vi "app - Kim Thing -- torque.vi"() -> ()   [LabVIEW 2012]
uses:
  <vilib>/event_ctls.llb/eventvkey.ctl
  cursor winow.ctl
  polynomial - bilinear.ctl
  torque transformation selector.ctl
  countdown control.ctl
  cursor window action.ctl
  hash action control.ctl
  container action.ctl
  array -- fit control .ctl
  cursor action.ctl
  fit function selector control.ctl
  file -- read-write control.ctl
  torque -- filename action.ctl
  torque -- hash key.ctl
panel:
  in  "torque transformations":T1
  out "offset (deg)":dbl
  out "sin2theta fit":dbl[](array[numeric])
  out "Plot: slope vs angle":cluster{dbl[], dbl[]}[](graph)
  in  "main folder":path=path "C:/Users/224586/Downloads/arkady/Torque-Jun2013"
  in  "Tab : other":enum32{"indicators", "other", "slope fit"}(tab)
  out "Torque (a.u)":dbl
  out "field (T)":dbl
  in  "angle":u16(ring) items=["-54", "-36", "-9", "27", "36", "45", "54"]
  in  "temperature":u16(ring) items=["2K", "15K", "30K", "38K", "42K", "45K", "52K", "60K", "75K", "90K", "100K", "120K", "150K", "180K", "240K"]
  out "time (sec)":dbl=513.2382892057026
  in  "open (o)":bool
  in  "plot (p)":bool
  out "temperature (K)":dbl=369.642
  out "angle (deg)":dbl
  in  "rotation set":u16(ring) items=["rotationset1", "rotationset2", "rotationset3", "rotationset4", "rotationset5", "rotationset6"]
  in  "filename":u16(ring) items=["5_60K_-54.dat", "5_60K_-36.dat", "5_60K_-9.dat", "5_60K_27.dat", "5_60K_36.dat", "5_60K_45.dat", "5_60K_54.dat"]
  out "read OK":bool=TRUE
  out "Char":i16=46
  out "VKey":T2
  in  "Tab: timer":enum32{"timer ON", "timer OFF"}(tab)=enum."timer OFF"
  in  "timer  \"update\"":dbl(slide) min=-553366660.0 max=2129711151.0 step=0.010000000000000002 scale=0.0..100.0 scale format="%#3_3f"
  out "folder --OK":bool=TRUE
  in  "temperatures":dbl[](array[numeric])
  in  "plot type":T3(ring)=enum."plot vs Temperature"
  out "current angle  index":dbl=1431.5698546544484
  out "current time index":dbl=1431.5698546544484
  in  "angles (deg)":dbl[](array[numeric])
  in  "slopes":dbl[](array[numeric])
  out "slope fit parameters":dbl[](array[numeric])
  out "field offset":dbl=1431.5698546544484
  out "torque offset":dbl=1431.5698546544484
  out "right bound index":dbl=1431.5698546544484
  out "left bound index":dbl=1431.5698546544484
  in  "Tab : all":enum32{"everything", "everything else"}(tab)
  out "Plot: torque/field -- all":cluster{dbl[], dbl[]}[](graph)
  out "Plot: temp vs time":cluster{dbl[], dbl[]}[](graph)
  out "Plot: torque --one angle":cluster{dbl[], dbl[]}[](graph)
  out "Plot: field vs time":cluster{dbl[], dbl[]}[](graph)
  out "Plot: torque -- all angles":cluster{dbl[], dbl[]}[](graph)
  in  "file path":path=path "C:/Data/GloveBox/Pu-delta-temperature_experiment/4_Sweep_370K_114.59min/9w/monitor/381_mo.dat"
  in  "cursor bracket: torque -- all angles":T4={"left"=364.687, "right "=367.23699999999997, "center"=365.962, "window"=2.5500000000000114, "cursors"=[1, 2, 3], "relative"=0, "absolute"=0, "fixed vertical offset"=0.0, "vertical offset"=0.0, "skew"=0.0, "default window frac"=0.1, "kind"=enum."symmetric", "skew.left"=0.5, "skew.right"=0.5, "Plot ref"=refnum, "wing order"=enum."forw"}
  in  "cursor bracket: field vs time":T4={"left"=295.7230142566191, "right "=904.2769857433809, "center"=600.0, "window"=608.5539714867618, "cursors"=[1, 2, 3], "relative"=2, "absolute"=3, "fixed vertical offset"=0.0, "vertical offset"=0.0, "skew"=0.0, "default window frac"=0.1, "kind"=enum."symmetric", "skew.left"=0.5, "skew.right"=0.5, "Plot ref"=refnum, "wing order"=enum."forw"}
  in  "temperature folder":path=path "C:/Data/GloveBox/Pu-delta-temperature_experiment"
  in  "rotation set folder":path=path "C:/Data/GloveBox/Pu-delta-temperature_experiment"
  in  "cursor bracket: torque/field -- all":T4={"left"=295.7230142566191, "right "=904.2769857433809, "center"=600.0, "window"=608.5539714867618, "cursors"=[1, 2, 3], "relative"=2, "absolute"=3, "fixed vertical offset"=0.0, "vertical offset"=0.0, "skew"=0.0, "default window frac"=0.1, "kind"=enum."symmetric", "skew.left"=0.5, "skew.right"=0.5, "Plot ref"=refnum, "wing order"=enum."forw"}
  in  "cursor bracket: torque -- one angle":T4={"left"=295.7230142566191, "right "=904.2769857433809, "center"=600.0, "window"=608.5539714867618, "cursors"=[1, 2, 3], "relative"=2, "absolute"=3, "fixed vertical offset"=0.0, "vertical offset"=0.0, "skew"=0.0, "default window frac"=0.1, "kind"=enum."symmetric", "skew.left"=0.5, "skew.right"=0.5, "Plot ref"=refnum, "wing order"=enum."forw"}
  out "sin2theta-fits":T5[](array[typedef])
  # "a sin( 2 x + b ) + c"
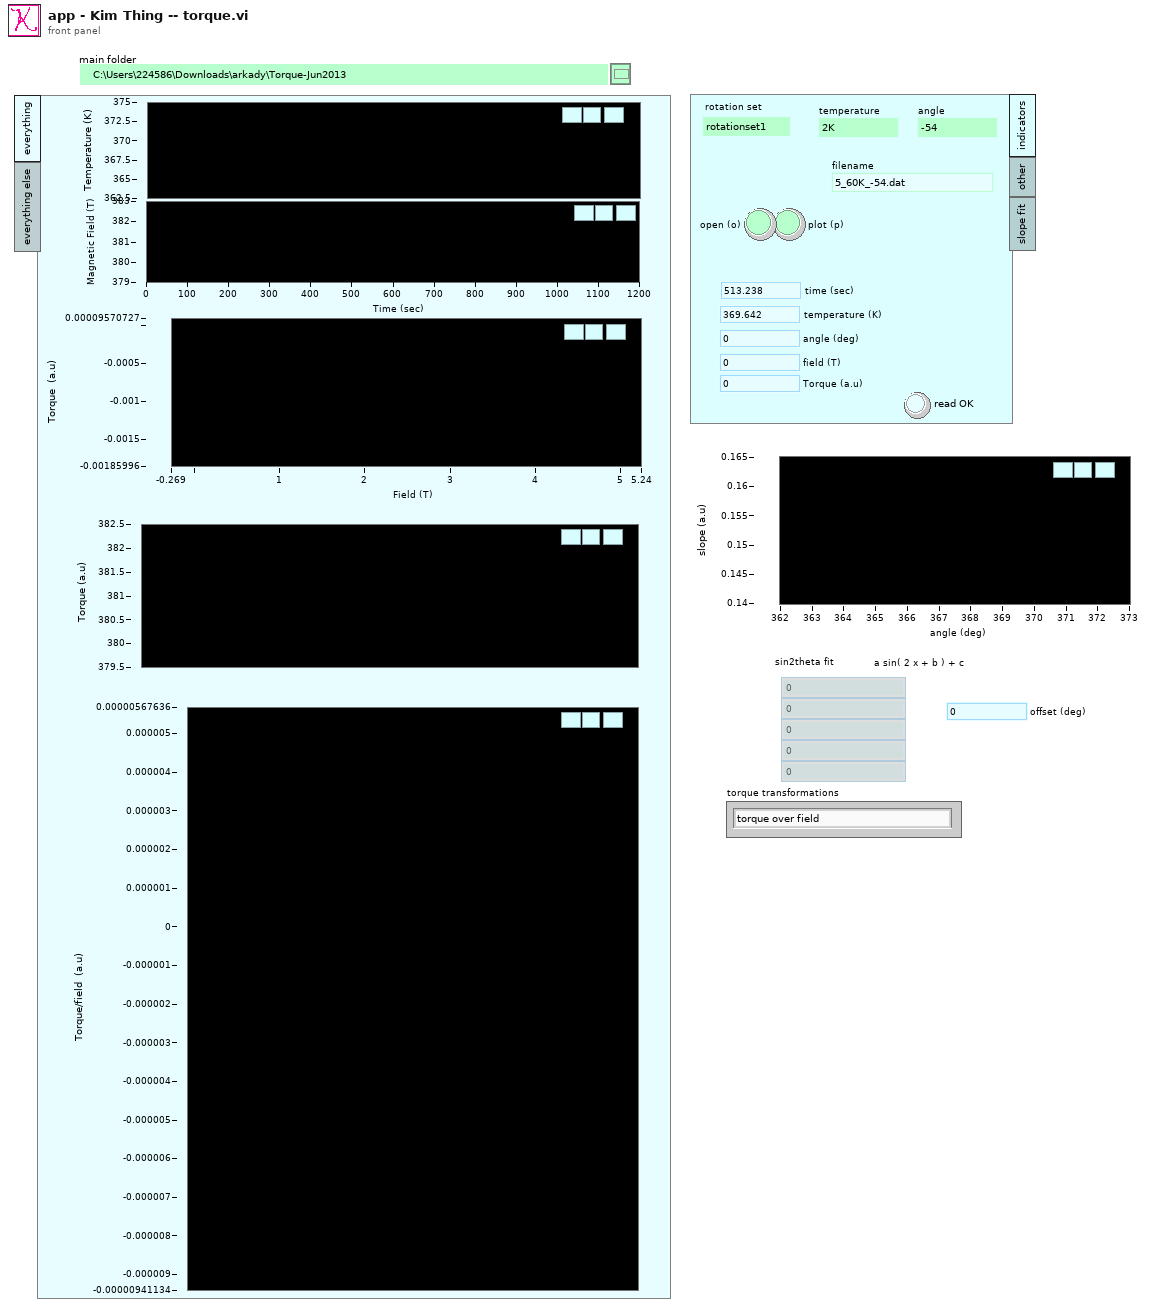
[diagram p1: front panel]
types:
  T1 = typedef "torque transformation selector.ctl" = enum16{"torque over field", "torque over field vs Hcos theta", "chi_torque vs Hcos theta"}
  T2 = typedef "eventvkey.ctl" = enum16{"ASCII", "Enter", "Return", "Shift", "Ctrl", "Alt", "Cmd", "Opt", "Caps", "NumLock", "Clear", "Break", "Up", "Down", "Left", "Right", "Insert", "Delete", "Home", "End", "PageUp", "PageDown", "Escape", "Help", "Pause", "ScrollLock", "F1", "F2", "F3", "F4", "F5", "F6", "F7", "F8", "F9", "F10", "F11", "F12", "F13", "F14", "F15", "F16", "F17", "F18", "F19", "F20", "F21", "F22", "F23", "F24", "Play", "VolumeUp", "VolumeDown", "Mute", "Two Byte Char"}
  T3 = enum16{"plot vs Magnetic Field", "plot vs Temperature"}
  T4 = typedef "cursor winow.ctl" = cluster{"left":dbl, "right ":dbl, "center":dbl, "window":dbl, "cursors":i32[], "relative":i32, "absolute":i32, "fixed vertical offset":dbl, "vertical offset":dbl, "skew":dbl, "default window frac":dbl, "kind":enum16{"symmetric", "skewed", "fancy"}, "skew.left":dbl, "skew.right":dbl, "Plot ref":refnum<vi>, "wing order":enum16{"forw", "back"}}
  T5 = typedef "polynomial - bilinear.ctl" = cluster{"a":dbl, "b":dbl, "c":dbl}
  T6 = typedef "cursor window action.ctl" = enum16{"balance", "h. offset change", "cursor moves", "change center", "change window", "init", "check", "reset", "set y to middle", "idle", "-write all Y", "-write left.X", "-write center.X", "-write right.X", "-write all X", "-change center", "-change window", "-change skew", "-read cursor 2", "-read cursor 1", "-read cursor 0", "-read all cursors", "-reset", "-read plot scale", "-set y to middle", "-Q: center.Y is visible", "-Q: window is visible", "-parse center.Y", "-right left from center", "-left move", "-right move", "-set center.Y", "-empty", "-set cursors to default", "-check", "-write center.Y", "-copy cursor 1", "-copy cursor 0", "-copy cursor 2", "move right", "move left", "shrink", "broaden", "skew up", "skew down", "-write plot scale", "zoom X", "change cen&win", "zoom to all data"}
  T7 = typedef "countdown control.ctl" = enum16{"check", "start", "reset cont", "stop", "reset once"}
  T8 = typedef "hash action control.ctl" = enum16{"get", "new", "--void", "delete", "delete all", "set", "--delete if exists", "--create if not there", "list keys", "index forw", "index back", "check", "index set", "find key"}
  T9 = typedef "torque -- filename action.ctl" = enum16{"parse", "build", "check"}
  T10 = typedef "container action.ctl" = enum16{"get", "read file", "plot", "init", "set"}
  T11 = typedef "file -- read-write control.ctl" = enum16{"read", "write all", "append one line"}
  T12 = typedef "torque -- hash key.ctl" = cluster{"temperature(K)":dbl, "angle(deg)":dbl}
  T13 = typedef "array -- fit control .ctl" = enum16{"fit", "calc", "check", "init"}
  T14 = typedef "cursor action.ctl" = enum16{"range", "read", "write", "check", "zoom out", "smart zoom out"}
  T15 = typedef "torque -- hash value.ctl" = cluster{"time (sec) array":dbl[], "temperature (K) array":dbl[], "SRS Vx (V) array":dbl[], "field (T) array":dbl[], "filename":string, "time OK?":bool, "temperature OK?":bool, "SRS OK?":bool, "FIELD OK?":bool}
  T16 = cluster{"field (T) array":dbl[], "SRS Vx (V) array":dbl[]}
  T17 = cluster{"time (sec) array":dbl[], "temperature (K) array":dbl[]}
  T18 = cluster{"time (sec) array":dbl[], "field (T) array":dbl[]}
  T19 = cluster{"field (T) array":dbl[], "SRS Vx (V) array":dbl[]}[]
  T20 = cluster{"time (sec) array":dbl[], "temperature (K) array":dbl[]}[]
  T21 = cluster{"time (sec) array":dbl[], "field (T) array":dbl[]}[]
  T22 = typedef "fit function selector control.ctl" = enum16{"linear", "varshni", "varshni5", "LogMinusT", "hyperbola", "einstein", "sine", "sine2theta", "cos2theta"}
  T23 = cluster{"field (T) array":dbl[], "y OUT":dbl[]}[]
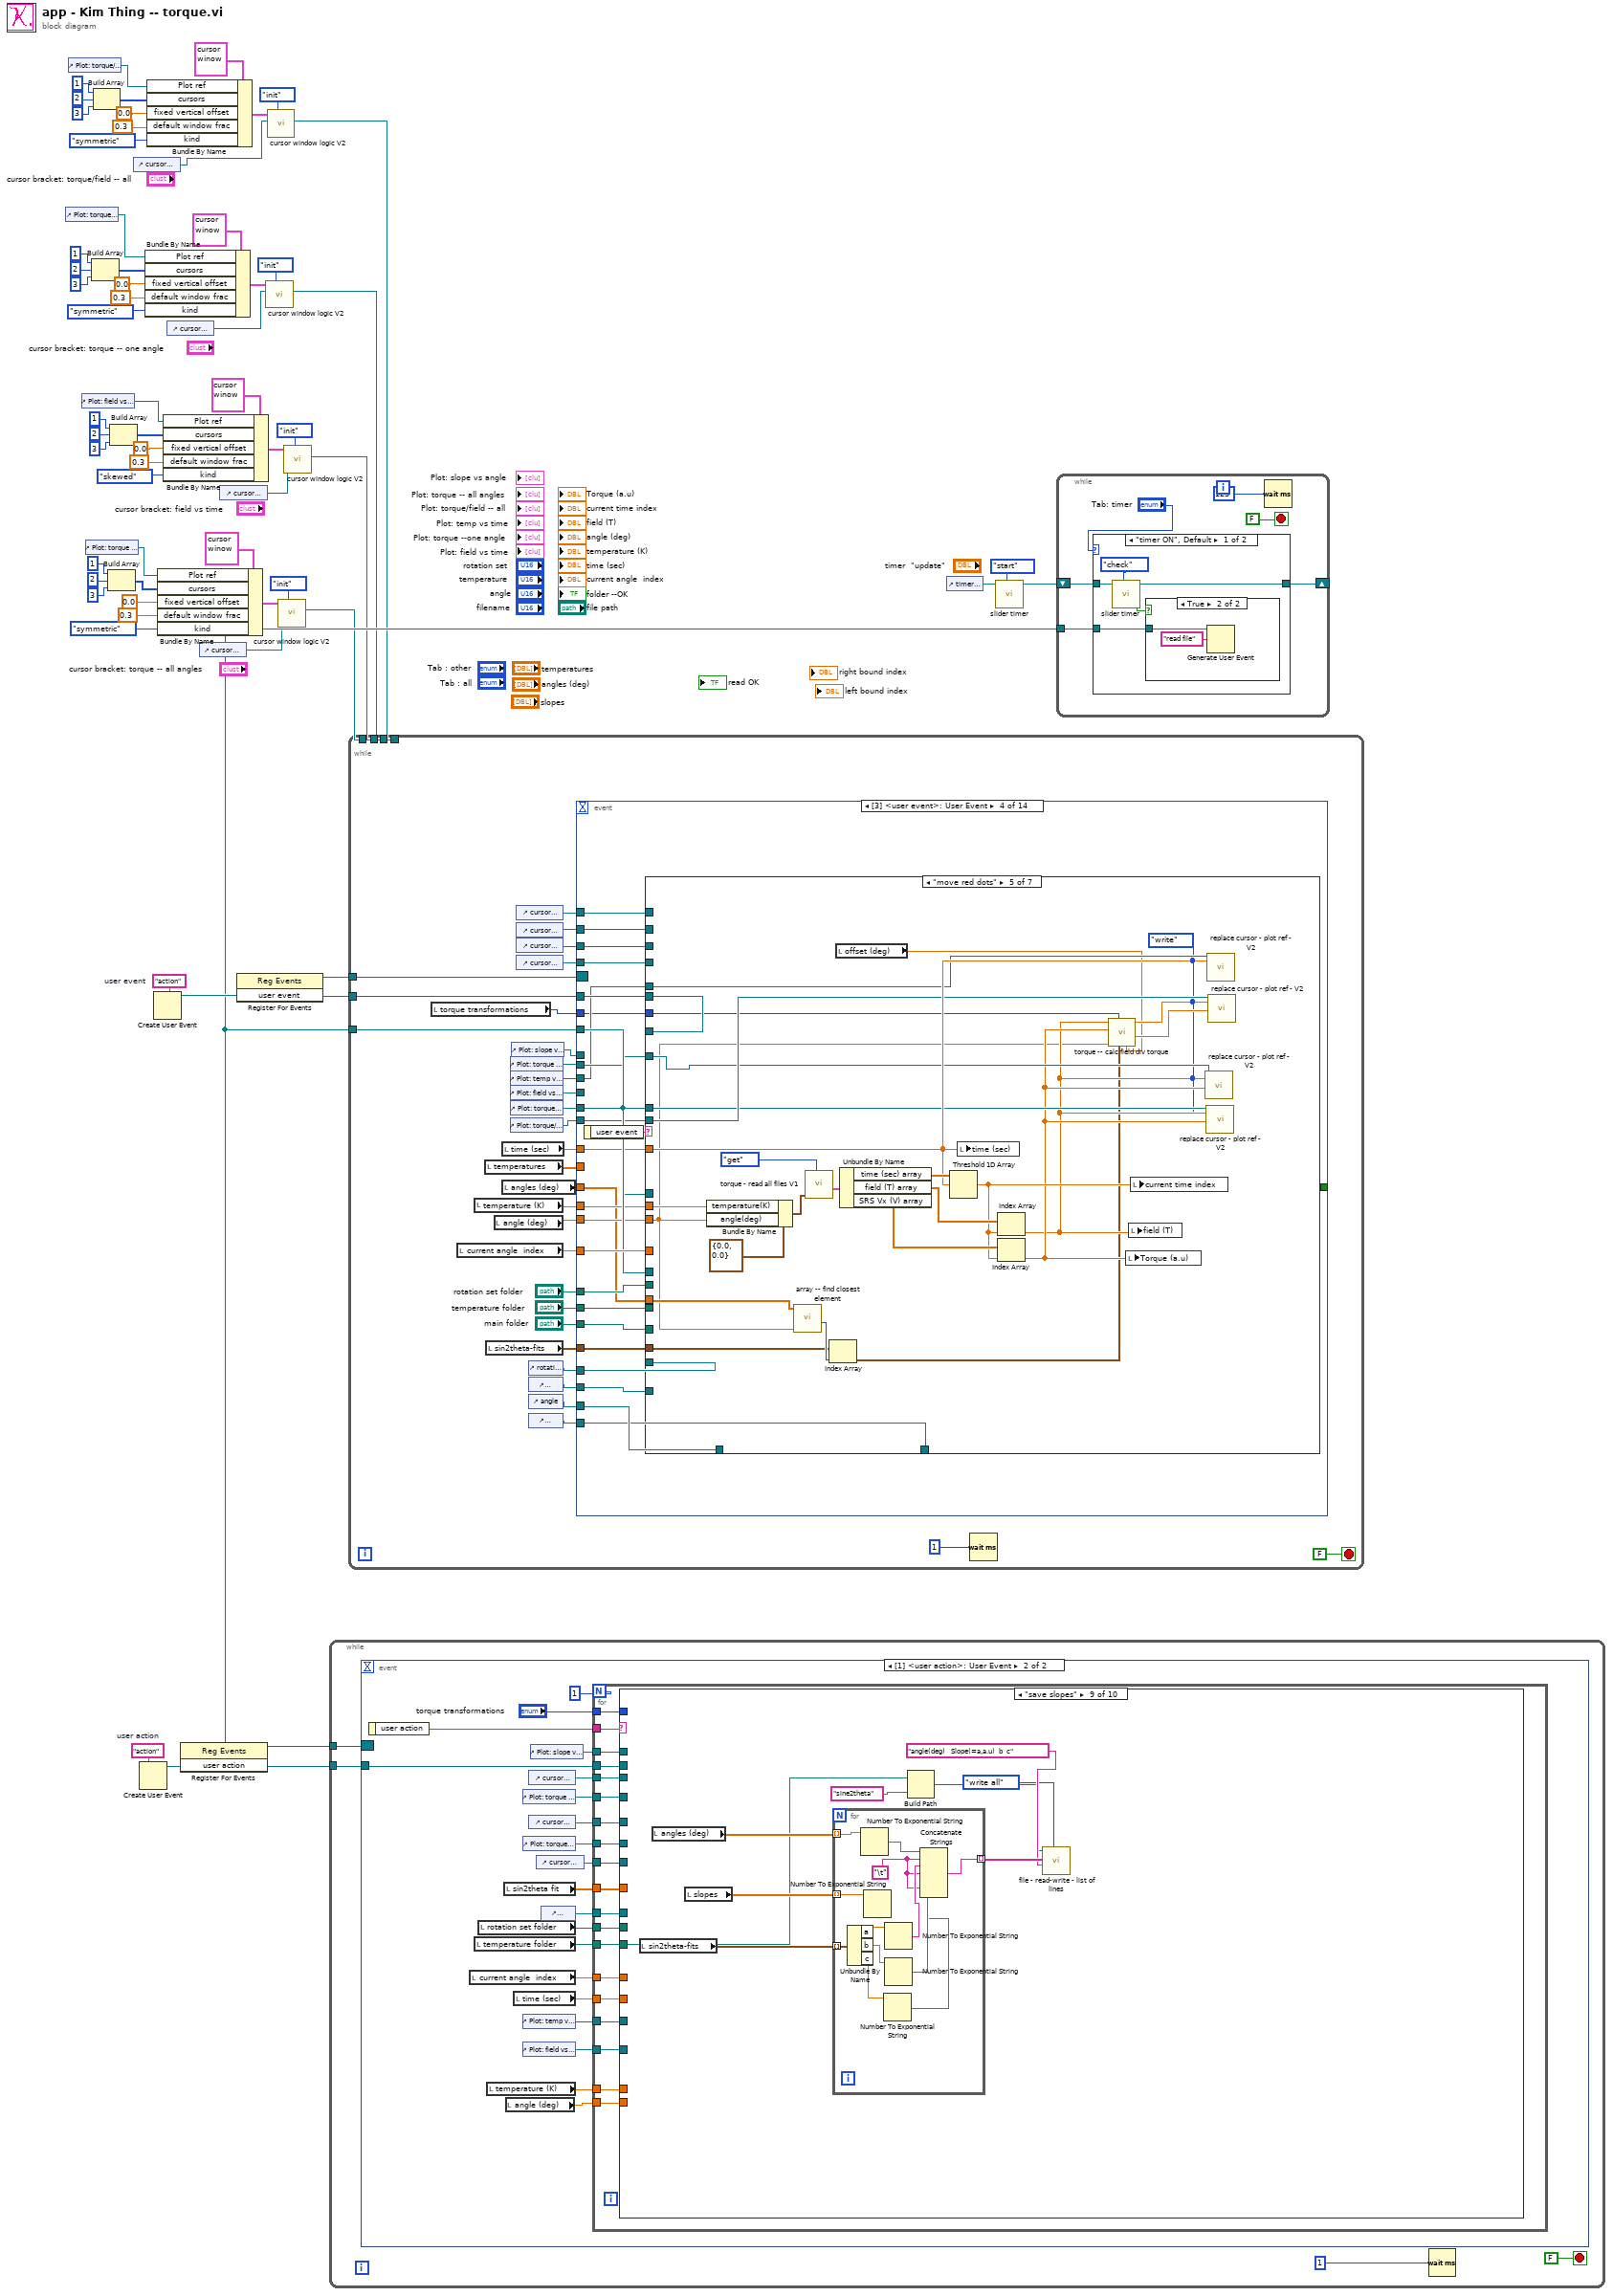
[diagram p0: block diagram]
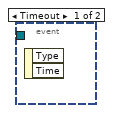
[diagram p4: hidden frame]
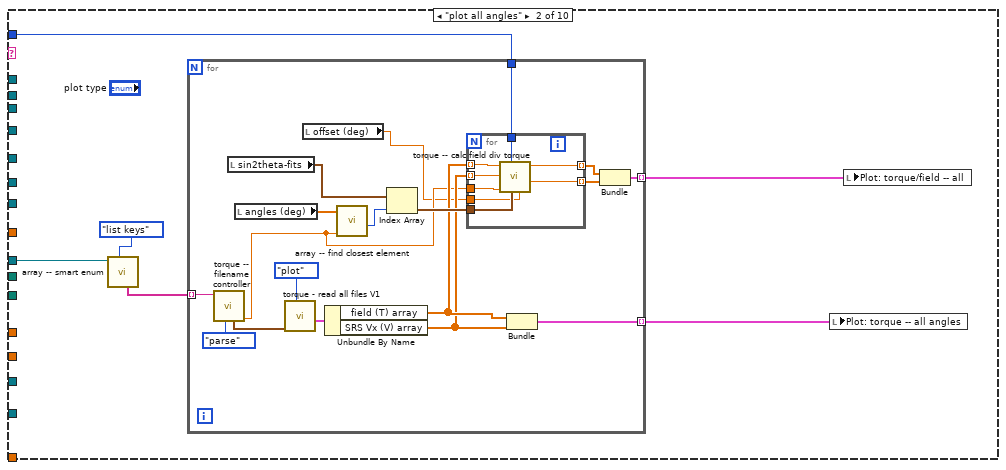
[diagram p6: hidden frame]
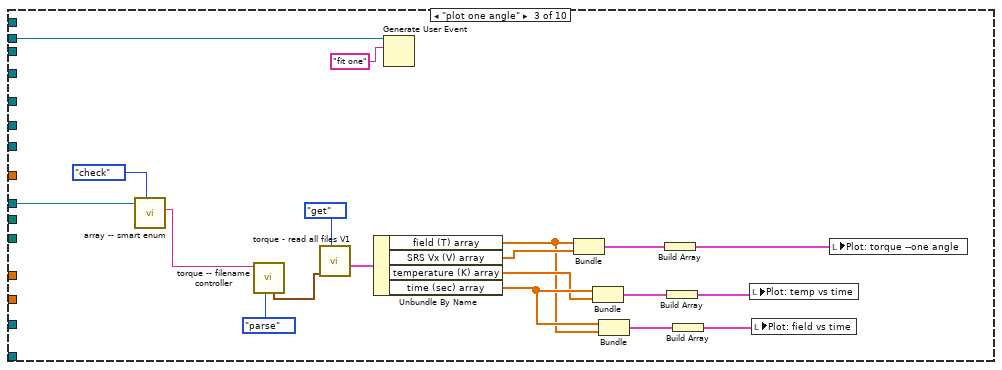
[diagram p7: hidden frame]
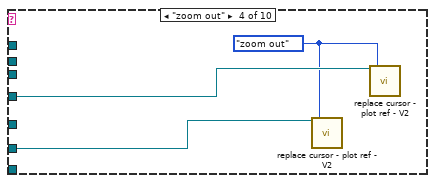
[diagram p8: hidden frame]
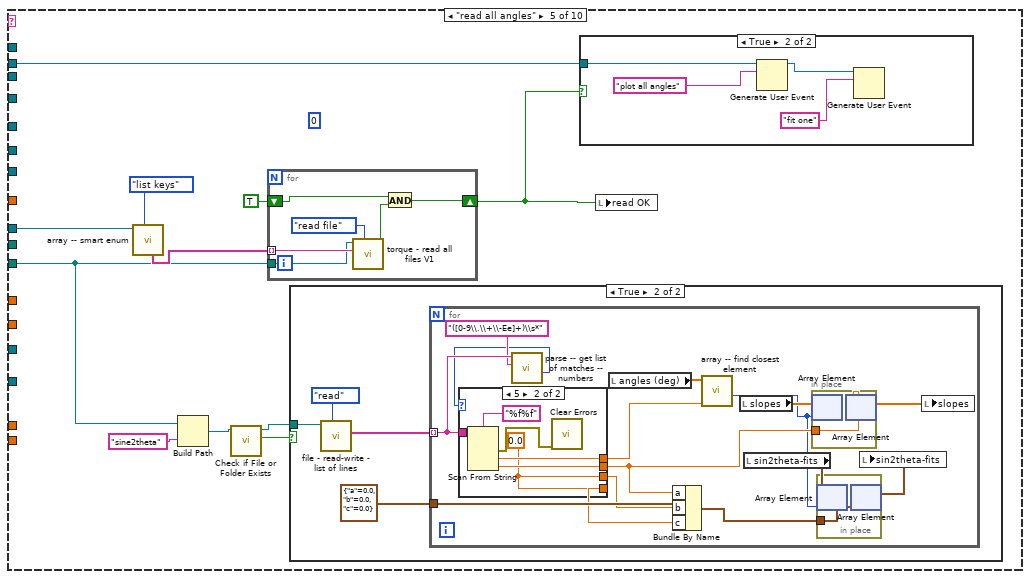
[diagram p9: hidden frame]
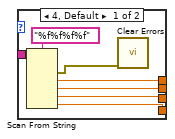
[diagram p11: hidden frame]
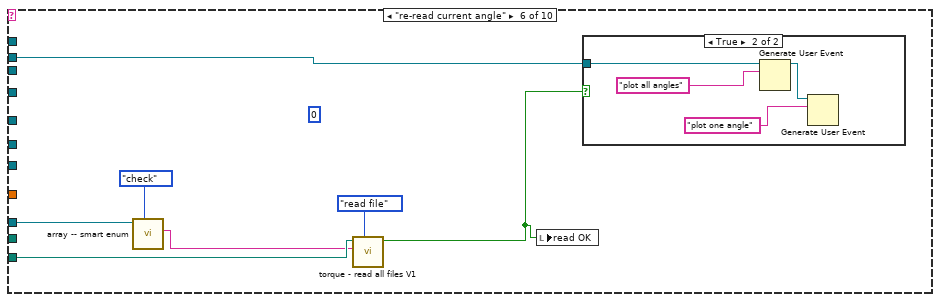
[diagram p13: hidden frame]
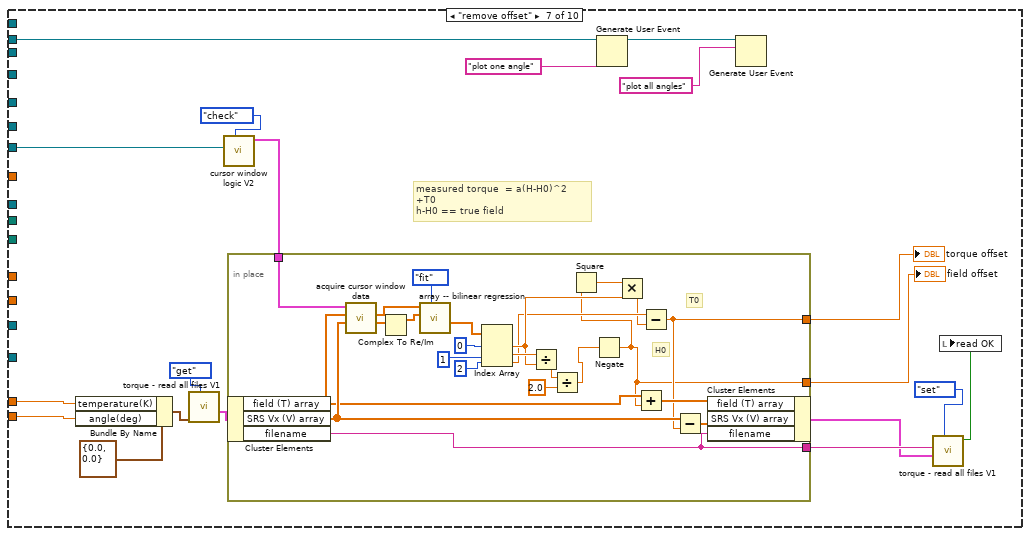
[diagram p15: hidden frame]
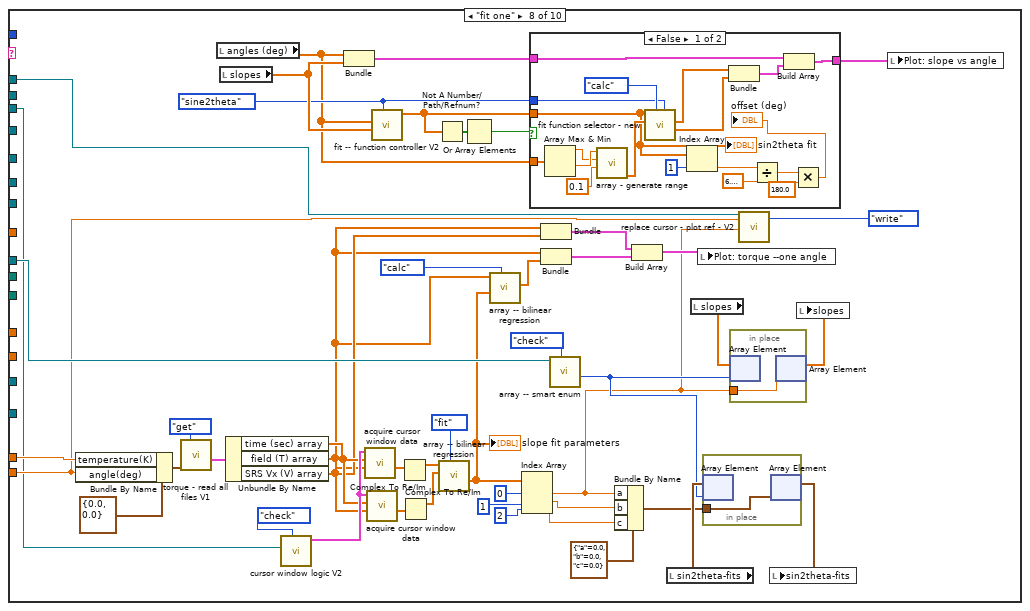
[diagram p16: hidden frame]
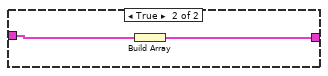
[diagram p17: hidden frame]
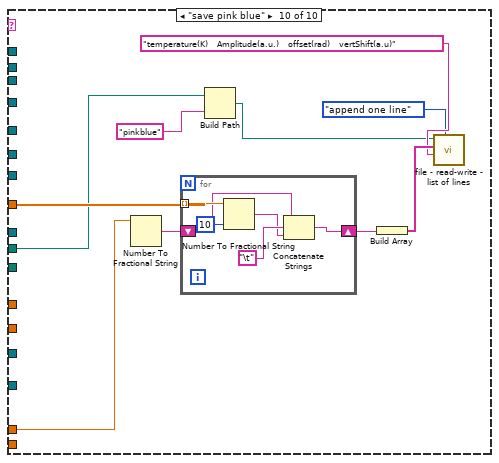
[diagram p18: hidden frame]
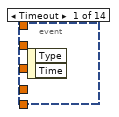
[diagram p19: hidden frame]
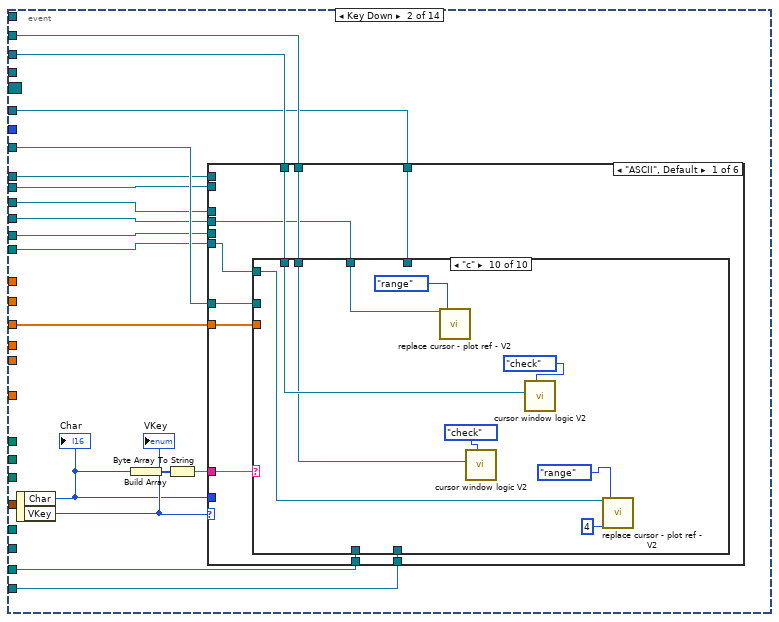
[diagram p20: hidden frame]
diagram:
  w58 = "action"  # user action
  w60 = "action"  # user event
  n1 = control-ref of="Plot: torque --one angle"() -> (w16:refnum<vi>)
  n2 = control-ref of="Plot: torque/field -- all"() -> (w2:refnum<vi>)
  n3 = control-ref of="Plot: field vs time"() -> (w32:refnum<vi>)
  n4 = control-ref of="Plot: torque -- all angles"() -> (w43:refnum<vi>)
  n5 = Build Array(1, 2, 3) -> (w17:i32[])
  n6 = Build Array(1, 2, 3) -> (w4:i32[])
  n7 = Build Array(1, 2, 3) -> (w28:i32[])
  n8 = Build Array(1, 2, 3) -> (w27:i32[])
  n9 = control-ref of="cursor bracket: torque/field -- all"() -> (w3:refnum<vi>)
  n10 = Create User Event(user event datatype=w58) -> (user event=w54:refnum<user-event>)  [unwired: 1 in, 1 out]
  n11 = Bundle By Name(cluster=T4 {"left"=0.0, "right "=0.0, "center"=0.0, "window"=0.0, "cursors"=[], "relative"=0, "absolute"=0, "fixed vertical offset"=0.0, "vertical offset"=0.0, "skew"=0.0, "default window frac"=0.0, "kind"=enum."symmetric", "skew.left"=0.0, "skew.right"=0.0, "Plot ref"=refnum, "wing order"=enum."forw"} ("cursor bracket in"), "Plot ref"=w16, "cursors"=w17, "fixed vertical offset"=0.0, "default window frac"=0.3 ("fixed vertical offset"), "kind"=enum16{"symmetric", "skewed", "fancy"}."symmetric") -> (w26:T4)
  n12 = Bundle By Name(cluster=T4 {"left"=0.0, "right "=0.0, "center"=0.0, "window"=0.0, "cursors"=[], "relative"=0, "absolute"=0, "fixed vertical offset"=0.0, "vertical offset"=0.0, "skew"=0.0, "default window frac"=0.0, "kind"=enum."symmetric", "skew.left"=0.0, "skew.right"=0.0, "Plot ref"=refnum, "wing order"=enum."forw"} ("cursor bracket in"), "Plot ref"=w2, "cursors"=w4, "fixed vertical offset"=0.0, "default window frac"=0.3 ("fixed vertical offset"), "kind"=enum16{"symmetric", "skewed", "fancy"}."symmetric") -> (w13:T4)
  n13 = Create User Event(user event datatype=w60) -> (user event=w57:refnum<user-event>)  [unwired: 1 in, 1 out]
  n14 = Bundle By Name(cluster=T4 {"left"=0.0, "right "=0.0, "center"=0.0, "window"=0.0, "cursors"=[], "relative"=0, "absolute"=0, "fixed vertical offset"=0.0, "vertical offset"=0.0, "skew"=0.0, "default window frac"=0.0, "kind"=enum."symmetric", "skew.left"=0.0, "skew.right"=0.0, "Plot ref"=refnum, "wing order"=enum."forw"} ("cursor bracket in"), "Plot ref"=w43, "cursors"=w28, "fixed vertical offset"=0.0, "default window frac"=0.3 ("fixed vertical offset"), "kind"=enum16{"symmetric", "skewed", "fancy"}."symmetric") -> (w52:T4)
  n15 = Bundle By Name(cluster=T4 {"left"=0.0, "right "=0.0, "center"=0.0, "window"=0.0, "cursors"=[], "relative"=0, "absolute"=0, "fixed vertical offset"=0.0, "vertical offset"=0.0, "skew"=0.0, "default window frac"=0.0, "kind"=enum."symmetric", "skew.left"=0.0, "skew.right"=0.0, "Plot ref"=refnum, "wing order"=enum."forw"} ("cursor bracket in"), "Plot ref"=w32, "cursors"=w27, "fixed vertical offset"=0.0, "default window frac"=0.3 ("fixed vertical offset"), "kind"=enum16{"symmetric", "skewed", "fancy"}."skewed") -> (w41:T4)
  n16 = control-ref of="cursor bracket: torque -- one angle"() -> (w15:refnum<vi>)
  n17 = register-events(w54) -> (reference out=w59:refnum<event-registration>)  [unwired: 2 in, 1 out]
  n18 = control-ref of="cursor bracket: torque -- all angles"() -> (w30:refnum<vi>)
  n19 = control-ref of="cursor bracket: field vs time"() -> (w29:refnum<vi>)
  n20 = register-events(w57) -> (reference out=w61:refnum<event-registration>)  [unwired: 2 in, 1 out]
  n21 = call "cursor window logic V2.vi"("cursor window action"=cursor_window_action."init", "cursor window in"=w15, "cursor window init"=w26) -> ("cursor window out"=w14:refnum<vi>)  [unwired: 7 in, 1 out]
  n22 = call "cursor window logic V2.vi"("cursor window action"=cursor_window_action."init", "cursor window in"=w3, "cursor window init"=w13) -> ("cursor window out"=w1:refnum<vi>)  [unwired: 7 in, 1 out]
  n23 = call "cursor window logic V2.vi"("cursor window action"=cursor_window_action."init", "cursor window in"=w30, "cursor window init"=w52) -> ("cursor window out"=w42:refnum<vi>)  [unwired: 7 in, 1 out]
  n24 = call "cursor window logic V2.vi"("cursor window action"=cursor_window_action."init", "cursor window in"=w29, "cursor window init"=w41) -> ("cursor window out"=w31:refnum<vi>)  [unwired: 7 in, 1 out]
  n25 = while {
    tunnel: w59 -> [w65]
    tunnel: w54 -> [w62]
    stop <- FALSE stop-if-true
    n26 = event shown="[1] <user action>: User Event" {
      selector: w65 -> [_ _]
      dyn-events: _ -> [_ _]
      timeout: _ -> [_ _]
      tunnel: w62 -> [_ w83]
      event Timeout {
        n27 = event-data() -> ()  [unwired: 1 in, 2 out]
      }
      event User Event {
        n28 = event-data() -> ("user action"=w85:string)  [unwired: 1 in]
        n29 = local read "current angle  index"() -> (w78:dbl)
        n30 = local read "temperature folder"() -> (w73:path)
        n31 = local read "rotation set folder"() -> (w67:path)
        n32 = local read "temperature (K)"() -> (w72:dbl)
        n33 = local read "sin2theta fit"() -> (w68:dbl[])
        n34 = local read "angle (deg)"() -> (w71:dbl)
        n35 = local read "time (sec)"() -> (w77:dbl)
        n36 = control-ref of="Plot: torque -- all angles"() -> (w81:refnum<vi>)
        n37 = control-ref of="Plot: torque --one angle"() -> (w82:refnum<vi>)
        n38 = control-ref of="Plot: temp vs time"() -> (w80:refnum<vi>)
        n39 = control-ref of="Plot: field vs time"() -> (w79:refnum<vi>)
        n40 = control-ref of="cursor bracket: temp vs time"() -> (w76:refnum<vi>)
        n41 = control-ref of="cursor bracket: torque/field -- all"() -> (w75:refnum<vi>)
        n42 = control-ref of="Plot: slope vs angle"() -> (w69:refnum<vi>)
        n43 = control-ref of="cursor bracket: torque -- one angle"() -> (w70:refnum<vi>)
        n44 = control-ref of="filename"() -> (w74:refnum<vi>)
        n45 = for {
          N: 1 -> [_]
          tunnel: w85 -> [w104]
          tunnel: w83 -> [w103]
          tunnel: w82 -> [w102]
          tunnel: w81 -> [w101]
          tunnel: w80 -> [w100]
          tunnel: w79 -> [w99]
          tunnel: w78 -> [w98]
          tunnel: w77 -> [w97]
          tunnel: w76 -> [w96]
          tunnel: w75 -> [w95]
          tunnel: w74 -> [w94]
          tunnel: w73 -> [w88]
          tunnel: w72 -> [w93]
          tunnel: w71 -> [w92]
          tunnel: w70 -> [w91]
          tunnel: w69 -> [w90]
          tunnel: w68 -> [w89]
          tunnel: w67 -> [w87]
          tunnel: "torque transformations" -> [w86]
          n46 = case shown="\"save slopes\"" w104 {
            tunnel: w103 -> [_ _ w137 _ w169 w220 w230 _ _ _]
            tunnel: w102 -> [_ _ _ w157 _ _ _ _ _ _]
            tunnel: w101 -> [_ _ _ w158 _ _ _ _ _ _]
            tunnel: w100 -> [_ _ _ _ _ _ _ _ _ _]
            tunnel: w99 -> [_ _ _ _ _ _ _ _ _ _]
            tunnel: w98 -> [_ _ _ _ _ _ _ _ _ _]
            tunnel: w97 -> [_ _ _ _ _ _ _ _ _ _]
            tunnel: w96 -> [_ _ _ _ _ _ _ w276 _ _]
            tunnel: w95 -> [_ _ _ _ _ _ _ _ _ _]
            tunnel: w94 -> [_ w107 w142 _ w167 w218 _ w304 _ _]
            tunnel: w88 -> [_ _ _ _ w163 w219 _ _ w345 _]
            tunnel: w93 -> [_ _ _ _ _ _ w241 w313 _ w366]
            tunnel: w92 -> [_ _ _ _ _ _ w240 w291 _ _]
            tunnel: w91 -> [_ _ _ _ _ _ w238 _ _ _]
            tunnel: w90 -> [_ _ _ _ _ _ _ w290 _ _]
            tunnel: w89 -> [_ _ _ _ _ _ _ _ _ w368]
            tunnel: w87 -> [_ _ _ _ _ _ _ _ _ w367]
            tunnel: w86 -> [_ w105 _ _ _ _ _ _ _ _]
            frame "False", Default {
            }
            frame "plot all angles" {
              n47 = call "array -- smart enum.vi"("hash action"=hash_action_control."list keys", "hash"=w107) -> ("Array of keys OUT"=w108:string[])  [unwired: 5 in, 4 out]
              n48 = for {
                tunnel: w108 -> [w126] mode=indexing
                tunnel: [w125] -> w110 mode=indexing
                tunnel: [w124] -> w109 mode=indexing
                tunnel: w105 -> [w114]
                n49 = call "torque -- filename controller.vi"("filename action"=torque_--_filename_action."parse", "String"=w126) -> ("Angle (deg)"=w112:dbl, "hash key"=w123:T12)  [unwired: 5 in, 3 out]
                n50 = local read "sin2theta-fits"() -> (w119:T5[])
                n51 = local read "angles (deg)"() -> (w121:dbl[])
                n52 = call "torque - read all files V1.vi"("container action"=container_action."plot", "hash key"=w123) -> ("torque -- hash value OUT"=w122:T15)  [unwired: 8 in, 1 out]
                n53 = local read "offset (deg)"() -> (w111:dbl)
                n54 = Unbundle By Name(w122) -> ("field (T) array"=w117:dbl[], "SRS Vx (V) array"=w116:dbl[])
                n55 = call "array -- find closest element.vi"("number"=w112, "Array"=w121) -> ("index"=w120:i32)  [unwired: 8 in, 1 out]
                n56 = Index Array(array=w119, index=w120) -> (element=w118:T5)
                n57 = for {
                  tunnel: w118 -> [w136]
                  tunnel: w117 -> [w135] mode=indexing
                  tunnel: w116 -> [w134] mode=indexing
                  tunnel: [w133] -> w115 mode=indexing
                  tunnel: w114 -> [w132]
                  tunnel: w112 -> [w130]
                  tunnel: [w131] -> w113 mode=indexing
                  tunnel: w111 -> [w129]
                  n58 = call "torque -- calc field div torque.vi"("angle offset"=w129, "parabola"=w136, "torque transformations"=w132, "angle"=w130, "torque"=w134, "field"=w135) -> ("transformed Y"=w133:dbl, "field out"=w131:dbl)  [unwired: 4 in]
                }
                n59 = Bundle("field (T) array"=w117, "SRS Vx (V) array"=w116) -> (w125:T16)  [unwired: 1 in]
                n60 = Bundle(w113, w115) -> (w124:cluster{dbl[], dbl[]})  [unwired: 1 in]
              }
              n61 = local write "Plot: torque -- all angles"(w110) -> ()
              n62 = local write "Plot: torque/field -- all"(w109) -> ()
            }
            frame "plot one angle" {
              n63 = call "array -- smart enum.vi"("hash action"=hash_action_control."check", "hash"=w142) -> ("hash key OUT"=w140:string)  [unwired: 5 in, 4 out]
              n64 = call "torque -- filename controller.vi"("filename action"=torque_--_filename_action."parse", "String"=w140) -> ("hash key"=w139:T12)  [unwired: 5 in, 4 out]
              n65 = call "torque - read all files V1.vi"("container action"=container_action."get", "hash key"=w139) -> ("torque -- hash value OUT"=w154:T15)  [unwired: 8 in, 1 out]
              n66 = Unbundle By Name(w154) -> ("field (T) array"=w143:dbl[], "SRS Vx (V) array"=w153:dbl[], "temperature (K) array"=w144:dbl[], "time (sec) array"=w147:dbl[])
              n67 = Generate User Event(user event=w137, event data cluster="fit one" ("event data")) -> ()  [unwired: 1 in, 2 out]
              n68 = Bundle("field (T) array"=w143, "SRS Vx (V) array"=w153) -> (w151:T16)  [unwired: 1 in]
              n69 = Bundle("time (sec) array"=w147, "temperature (K) array"=w144) -> (w149:T17)  [unwired: 1 in]
              n70 = Bundle("time (sec) array"=w147, "field (T) array"=w143) -> (w148:T18)  [unwired: 1 in]
              n71 = Build Array(w151) -> (w150:T19)
              n72 = Build Array(w149) -> (w145:T20)
              n73 = Build Array(w148) -> (w146:T21)
              n74 = local write "Plot: temp vs time"(w145) -> ()
              n75 = local write "Plot: field vs time"(w146) -> ()
              n76 = local write "Plot: torque --one angle"(w150) -> ()
            }
            frame "zoom out" {
              w156 = cursor_action."zoom out" ("cursor action")
              n77 = call "replace cursor - plot ref - V2.vi"("Plot ref in"=w157, "cursor action"=w156) -> ()  [unwired: 15 in, 3 out]
              n78 = call "replace cursor - plot ref - V2.vi"("Plot ref in"=w158, "cursor action"=w156) -> ()  [unwired: 15 in, 3 out]
            }
            frame "read all angles" {
              (unwired) 0 ("Numeric Control")
              n79 = call "array -- smart enum.vi"("hash action"=hash_action_control."list keys", "hash"=w167) -> ("Array of keys OUT"=w165:string[])  [unwired: 5 in, 4 out]
              n80 = Build Path(base path=w163, name or relative path="sine2theta") -> (appended path=w161:path)
              n81 = call <vilib>:"Check if File or Folder Exists.vi"("path"=w161) -> ("file or folder exists?"=w160:bool, "dup path"=w159:path)  [unwired: 8 in, 1 out]
              n82 = for {
                tunnel: w165 -> [w209] mode=indexing
                tunnel: w163 -> [w208]
                shift-right: [w207] -> w164
                shift-left: TRUE -> [w206]
                n83 = call "torque - read all files V1.vi"("container action"=container_action."read file", "filename"=w209, "folder Path"=w208) -> ("OK?"=w205:bool)  [unwired: 7 in, 1 out]
                n84 = And(x=w206, y=w205) -> (x .and. y?=w207:bool)
              }
              n85 = case shown="True" w160 {
                tunnel: w159 -> [_ w173]
                frame False {
                }
                frame True {
                  n86 = call "file - read-write - list of lines.vi"("read/write control"=file_--_read-write_control."read", "file path"=w173) -> ("list of lines OUT"=w171:string[])  [unwired: 8 in, 1 out]
                  n87 = for {
                    tunnel: w171 -> [w176] mode=indexing
                    tunnel: T5 {"a"=0.0, "b"=0.0, "c"=0.0} ("parabola") -> [w184]
                    n88 = call "parse -- get list of matches -- numbers.vi"("regexp"="([0-9\\.\\+\\-Ee]+)\\s*", "string"=w176) -> ("# of numbers"=w174:i32)  [unwired: 6 in, 3 out]
                    n89 = case shown="5" w174 {
                      tunnel: [w194 w200] -> w185
                      tunnel: [w193 w199] -> w183
                      tunnel: [w192 w197] -> w182
                      tunnel: [w191 w197] -> w181
                      tunnel: w176 -> [w190 w198]
                      frame 4, Default {
                        n90 = Scan From String(format string="%f%f%f%f", input string=w190) -> (error out=w189:errorcluster, output 1=w194:dbl, output 2=w193:dbl, output 3=w192:dbl, output 4=w191:dbl)  [unwired: 6 in, 2 out]
                        n91 = call <vilib>:"Clear Errors.vi"("error in (no error)"=w189) -> ()  [unwired: 6 in, 1 out]
                      }
                      frame 5 {
                        w197 = 0.0
                        n92 = Scan From String(format string="%f%f", input string=w198) -> (error out=w196:errorcluster, output 1=w200:dbl, output 2=w199:dbl)  [unwired: 4 in, 2 out]
                        n93 = call <vilib>:"Clear Errors.vi"("error in (no error)"=w196) -> ()  [unwired: 6 in, 1 out]
                      }
                    }
                    n94 = local read "angles (deg)"() -> (w186:dbl[])
                    n95 = Bundle By Name(cluster=w184, "a"=w183, "b"=w182, "c"=w181) -> (w179:T5)
                    n96 = call "array -- find closest element.vi"("number"=w185, "Array"=w186) -> ("index"=w177:i32)  [unwired: 8 in, 1 out]
                    n97 = local read "slopes"() -> (w188:dbl[])
                    n98 = local read "sin2theta-fits"() -> (w180:T5[])
                    n99 = in-place {
                      in-place-border: w183 -> [w203]
                      n100 = in-place-array #1(w188, w177) -> ()  [unwired: 1 out]
                      n101 = in-place-array #1(w203) -> (w187:dbl[])  [unwired: 1 out]
                    }
                    n102 = in-place {
                      in-place-border: w179 -> [w202]
                      n103 = in-place-array #2(w180, w177) -> ()  [unwired: 1 out]
                      n104 = in-place-array #2(w202) -> (w178:T5[])  [unwired: 1 out]
                    }
                    n105 = local write "sin2theta-fits"(w178) -> ()
                    n106 = local write "slopes"(w187) -> ()
                  }
                }
              }
              n107 = case shown="True" w164 {
                tunnel: w169 -> [_ w212]
                frame False {
                }
                frame True {
                  n108 = Generate User Event(user event=w212, event data cluster="plot all angles" ("event data")) -> (user event out=w211:refnum<user-event>)  [unwired: 1 in, 1 out]
                  n109 = Generate User Event(user event=w211, event data cluster="fit one" ("event data")) -> ()  [unwired: 1 in, 2 out]
                }
              }
              n110 = local write "read OK"(w164) -> ()
            }
            frame "re-read current angle" {
              (unwired) 0 ("Numeric Control")
              n111 = call "array -- smart enum.vi"("hash action"=hash_action_control."check", "hash"=w218) -> ("hash key OUT"=w215:string)  [unwired: 5 in, 4 out]
              n112 = call "torque - read all files V1.vi"("container action"=container_action."read file", "filename"=w215, "folder Path"=w219) -> ("OK?"=w214:bool)  [unwired: 7 in, 1 out]
              n113 = local write "read OK"(w214) -> ()
              n114 = case shown="True" w214 {
                tunnel: w220 -> [_ w223]
                frame False {
                }
                frame True {
                  n115 = Generate User Event(user event=w223, event data cluster="plot all angles" ("event data")) -> (user event out=w222:refnum<user-event>)  [unwired: 1 in, 1 out]
                  n116 = Generate User Event(user event=w222, event data cluster="plot one angle" ("event data")) -> ()  [unwired: 1 in, 2 out]
                }
              }
            }
            frame "remove offset" {
              # "measured torque  = a(H-H0)^2 +T0\nh-H0 == true field"
              n117 = Bundle By Name(cluster=T12 {"temperature(K)"=0.0, "angle(deg)"=0.0} ("hash key"), "temperature(K)"=w241, "angle(deg)"=w240) -> (w235:T12)
              n118 = call "torque - read all files V1.vi"("container action"=container_action."get", "hash key"=w235) -> ("torque -- hash value OUT"=w239:T15)  [unwired: 8 in, 1 out]
              n119 = call "cursor window logic V2.vi"("cursor window action"=cursor_window_action."check", "cursor window in"=w238) -> ("cursor window out"=w236:T4)  [unwired: 8 in, 1 out]
              n120 = in-place {
                in-place-border: w236 -> [w266]
                in-place-border: [w247] -> w234
                in-place-border: [w244] -> w227
                in-place-border: [w246] -> w226
                # "T0"
                # "H0"
                n121 = in-place-cluster #3(w239) -> ("field (T) array"=w249:dbl[], "SRS Vx (V) array"=w251:dbl[], "filename"=w247:string)
                n122 = call "acquire cursor window data.vi"("z in"=w251, "omega in"=w249, "cursor window"=w266) -> ("z out"=w264:cdb[], "omega  out"=w265:dbl[])  [unwired: 4 in, 3 out]
                n123 = Complex To Re/Im(x + iy=w264) -> (x=w263:dbl[])  [unwired: 1 out]
                n124 = call "array -- bilinear regression.vi"("action"=array_--_fit_control_."fit", "y"=w263, "x"=w265) -> ("fit OUT"=w262:dbl[])  [unwired: 6 in, 2 out]
                n125 = Index Array(array=w262, index #1=0 ("index"), index #2=1 ("index"), index #3=2 ("index")) -> (element #1=w254:dbl, element #2=w258:dbl, element #3=w253:dbl)
                n126 = Divide(x=w258, y=w254) -> (x/y=w257:dbl)
                n127 = Divide(x=w257, y=2.0) -> (x/y=w245:dbl)
                n128 = Negate(x=w245) -> (-x=w244:dbl)
                n129 = Square(x=w244) -> (x^2=w255:dbl)
                n130 = Multiply(x=w255, y=w254) -> (x*y=w252:dbl)
                n131 = Add(x=w249, y=w244) -> (x+y=w248:dbl[])
                n132 = Subtract(x=w253, y=w252) -> (x-y=w246:dbl)
                n133 = Subtract(x=w251, y=w246) -> (x-y=w250:dbl[])
                n134 = in-place-cluster #3("field (T) array"=w248, "SRS Vx (V) array"=w250, "filename"=w247) -> (w232:T15)
              }
              "field offset" <- w227
              "torque offset" <- w226
              n135 = Generate User Event(user event=w230, event data cluster="plot one angle" ("event data")) -> (user event out=w229:refnum<user-event>)  [unwired: 1 in, 1 out]
              n136 = Generate User Event(user event=w229, event data cluster="plot all angles" ("event data")) -> ()  [unwired: 1 in, 2 out]
              n137 = call "torque - read all files V1.vi"("container action"=container_action."set", "torque -- hash value IN"=w232, "filename"=w234) -> ("OK?"=w225:bool)  [unwired: 7 in, 1 out]
              n138 = local write "read OK"(w225) -> ()
            }
            frame "fit one" {
              w288 = fit_function_selector_control."sine2theta" ("fit using")
              n139 = Bundle By Name(cluster=T12 {"temperature(K)"=0.0, "angle(deg)"=0.0} ("hash key"), "temperature(K)"=w313, "angle(deg)"=w291) -> (w310:T12)
              n140 = call "torque - read all files V1.vi"("container action"=container_action."get", "hash key"=w310) -> ("torque -- hash value OUT"=w312:T15)  [unwired: 8 in, 1 out]
              n141 = local read "angles (deg)"() -> (w287:dbl[])
              n142 = local read "slopes"() -> (w289:dbl[])
              n143 = Unbundle By Name(w312) -> ("time (sec) array"=w282:dbl[], "field (T) array"=w280:dbl[], "SRS Vx (V) array"=w281:dbl[])
              n144 = call "cursor window logic V2.vi"("cursor window action"=cursor_window_action."check", "cursor window in"=w276) -> ("cursor window out"=w283:T4)  [unwired: 8 in, 1 out]
              n145 = Bundle("angles (deg)"=w287, "slopes"=w289) -> (w294:cluster{"angles (deg)":dbl[], "slopes":dbl[]})  [unwired: 1 in]
              n146 = call "acquire cursor window data.vi"("z in"=w280, "omega in"=w282, "cursor window"=w283) -> ("z out"=w308:cdb[])  [unwired: 4 in, 4 out]
              n147 = call "acquire cursor window data.vi"("z in"=w281, "omega in"=w282, "cursor window"=w283) -> ("z out"=w279:cdb[])  [unwired: 4 in, 4 out]
              n148 = call "fit -- function controller V2.vi"("fit using"=w288, "y"=w289, "x"=w287) -> ("best fit parameters"=w286:dbl[])  [unwired: 8 in]
              n149 = Complex To Re/Im(x + iy=w308) -> (x=w278:dbl[])  [unwired: 1 out]
              n150 = Complex To Re/Im(x + iy=w279) -> (x=w277:dbl[])  [unwired: 1 out]
              n151 = Not A Number/Path/Refnum?(number/path/refnum=w286) -> (NaN/Path/Refnum?=w285:bool[])
              n152 = call "array -- bilinear regression.vi"("action"=array_--_fit_control_."fit", "y"=w277, "x"=w278) -> ("fit OUT"=w295:dbl[])  [unwired: 6 in, 2 out]
              "slope fit parameters" <- w295
              n153 = Or Array Elements(Boolean array=w285) -> (logical OR=w284:bool)
              n154 = call "array -- bilinear regression.vi"("action"=array_--_fit_control_."calc", "fit"=w295, "x"=w280) -> ("y OUT"=w297:dbl[])  [unwired: 6 in, 2 out]
              n155 = Index Array(array=w295, index #1=0 ("index"), index #2=1 ("index"), index #3=2 ("index")) -> (element #1=w270:dbl, element #2=w269:dbl, element #3=w268:dbl)
              n156 = case shown="False" w284 {
                tunnel: w294 -> [w335 w337]
                tunnel: [w334 w336] -> w293
                tunnel: w288 -> [w332 _]
                tunnel: w287 -> [w328 _]
                tunnel: w286 -> [w323 _]
                frame False {
                  n157 = Array Max & Min(array=w328) -> (max value=w326:dbl, min value=w327:dbl)  [unwired: 2 out]
                  n158 = call "array - generate range.vi"("df"=0.1, "freq max"=w326, "freq min"=w327) -> ("Array"=w324:dbl[])  [unwired: 7 in, 1 out]
                  n159 = call "fit function selector - new.vi"("fit using"=w332, "fit action"=array_--_fit_control_."calc", "x"=w324, "fit parameters"=w323) -> ("y out"=w330:dbl[], "x out"=w331:dbl[])  [unwired: 3 in, 3 out]
                  n160 = Index Array(array=w323, index=1) -> (element=w321:dbl)
                  n161 = Bundle("x out"=w331, "y out"=w330) -> (w329:cluster{"x out":dbl[], "y out":dbl[]})  [unwired: 1 in]
                  n162 = Divide(x=w321, y=6.283185307179586) -> (x/y=w319:dbl)
                  n163 = Build Array(w335, w329) -> (w334:cluster{"x out":dbl[], "y out":dbl[]}[])
                  n164 = Multiply(x=w319, y=180.0) -> (x*y=→"offset (deg)":dbl)
                  "sin2theta fit" <- w323
                }
                frame True {
                  n165 = Build Array(w337) -> (w336:cluster{"angles (deg)":dbl[], "slopes":dbl[]}[])
                }
              }
              n166 = Bundle("field (T) array"=w280, "SRS Vx (V) array"=w281) -> (w296:T16)  [unwired: 1 in]
              n167 = Bundle("field (T) array"=w280, "y OUT"=w297) -> (w300:cluster{"field (T) array":dbl[], "y OUT":dbl[]})  [unwired: 1 in]
              n168 = call "array -- smart enum.vi"("hash action"=hash_action_control."check", "hash"=w304) -> ("index OUT"=w273:i32)  [unwired: 5 in, 4 out]
              n169 = Bundle By Name(cluster=T5 {"a"=0.0, "b"=0.0, "c"=0.0} ("parabola"), "a"=w270, "b"=w269, "c"=w268) -> (w272:T5)
              n170 = Build Array(w296, w300) -> (w299:T23)
              n171 = local read "sin2theta-fits"() -> (w274:T5[])
              n172 = local read "slopes"() -> (w302:dbl[])
              n173 = local write "Plot: torque --one angle"(w299) -> ()
              n174 = in-place {
                in-place-border: w272 -> [w316]
                n175 = in-place-array #4(w274, w273) -> ()  [unwired: 1 out]
                n176 = in-place-array #4(w316) -> (w271:T5[])  [unwired: 1 out]
              }
              n177 = in-place {
                in-place-border: w270 -> [w338]
                n178 = in-place-array #5(w302, w273) -> ()  [unwired: 1 out]
                n179 = in-place-array #5(w338) -> (w301:dbl[])  [unwired: 1 out]
              }
              n180 = call "replace cursor - plot ref - V2.vi"("Plot ref in"=w290, "new X"=w291, "new  Y"=w270, "cursor action"=cursor_action."write") -> ()  [unwired: 13 in, 3 out]
              n181 = local write "sin2theta-fits"(w271) -> ()
              n182 = local write "slopes"(w301) -> ()
              n183 = local write "Plot: slope vs angle"(w293) -> ()
            }
            frame "save slopes" {
              n184 = local read "sin2theta-fits"() -> (w339:T5[])
              n185 = local read "angles (deg)"() -> (w347:dbl[])
              n186 = local read "slopes"() -> (w346:dbl[])
              n187 = for {
                tunnel: w347 -> [w359] mode=indexing
                tunnel: w346 -> [w358] mode=indexing
                tunnel: [w356] -> w343 mode=indexing
                tunnel: w339 -> [w355] mode=indexing
                w349 = "\t"
                n188 = Unbundle By Name(w355) -> ("a"=w354:dbl, "b"=w353:dbl, "c"=w352:dbl)
                n189 = Number To Exponential String(number=w359) -> (E-format string=w357:string)  [unwired: 3 in]
                n190 = Number To Exponential String(number=w358) -> ()  [unwired: 3 in, 1 out]
                n191 = Number To Exponential String(number=w352) -> (E-format string=w348:string)  [unwired: 3 in]
                n192 = Number To Exponential String(number=w354) -> (E-format string=w351:string)  [unwired: 3 in]
                n193 = Number To Exponential String(number=w353) -> (E-format string=w350:string)  [unwired: 3 in]
                n194 = Concatenate Strings(w357, w349, w351, w349, w350, w349, w348) -> (w356:string)
              }
              n195 = Build Path(base path=w345, name or relative path="sine2theta") -> (appended path=w341:path)
              n196 = call "file - read-write - list of lines.vi"("read/write control"=file_--_read-write_control."write all", "header"="angle(deg)   Slope(=a,a.u)  b  c" ("name or relative path"), "list of lines IN"=w343, "file path"=w341) -> ()  [unwired: 6 in, 2 out]
            }
            frame "save pink blue" {
              n197 = Number To Fractional String(number=w366) -> (F-format string=w365:string)  [unwired: 3 in]
              n198 = for {
                tunnel: w368 -> [w375] mode=indexing
                shift-right: [w374] -> w364
                shift-left: w365 -> [w371]
                n199 = Number To Fractional String(number=w375, precision (6)=i16 10) -> (F-format string=w372:string)  [unwired: 2 in]
                n200 = Concatenate Strings(w371, "\t", w372) -> (w374:string)
              }
              n201 = Build Path(base path=w367, name or relative path="pinkblue") -> (appended path=w361:path)
              n202 = Build Array(w364) -> (w363:string[])
              n203 = call "file - read-write - list of lines.vi"("read/write control"=file_--_read-write_control."append one line", "header"="temperature(K)   Amplitude(a.u.)   offset(rad)   vertShift(a.u)" ("name or relative path"), "list of lines IN"=w363, "file path"=w361) -> ()  [unwired: 6 in, 2 out]
            }
          }
        }
      }
    }
    n204 = Wait (ms)(milliseconds to wait=u32 1) -> ()  [unwired: 1 out]
  }
  n205 = while {
    tunnel: w61 -> [w405]
    tunnel: w54 -> [w402]
    tunnel: w57 -> [w398]
    tunnel: w42 -> [_]
    tunnel: w31 -> [_]
    tunnel: w14 -> [_]
    tunnel: w1 -> [_]
    stop <- FALSE stop-if-true
    n206 = local read "torque transformations"() -> (w377:T1)
    n207 = local read "current angle  index"() -> (w396:dbl)
    n208 = local read "temperature (K)"() -> (w383:dbl)
    n209 = local read "temperatures"() -> (w384:dbl[])
    n210 = local read "sin2theta-fits"() -> (w376:T5[])
    n211 = local read "angle (deg)"() -> (w382:dbl)
    n212 = local read "time (sec)"() -> (w378:dbl)
    n213 = local read "angles (deg)"() -> (w385:dbl[])
    n214 = control-ref of="Plot: torque -- all angles"() -> (w400:refnum<vi>)
    n215 = control-ref of="Plot: temp vs time"() -> (w397:refnum<vi>)
    n216 = control-ref of="Plot: field vs time"() -> (w401:refnum<vi>)
    n217 = control-ref of="Plot: torque --one angle"() -> (w399:refnum<vi>)
    n218 = control-ref of="Plot: torque/field -- all"() -> (w386:refnum<vi>)
    n219 = control-ref of="Plot: slope vs angle"() -> (w379:refnum<vi>)
    n220 = control-ref of="cursor bracket: torque/field -- all"() -> (w381:refnum<vi>)
    n221 = control-ref of="cursor bracket: field vs time"() -> (w393:refnum<vi>)
    n222 = control-ref of="cursor bracket: torque -- all angles"() -> (w392:refnum<vi>)
    n223 = control-ref of="cursor bracket: torque -- one angle"() -> (w380:refnum<vi>)
    n224 = control-ref of="rotation set"() -> (w394:refnum<vi>)
    n225 = control-ref of="temperature"() -> (w390:refnum<vi>)
    n226 = control-ref of="angle"() -> (w388:refnum<vi>)
    n227 = control-ref of="filename"() -> (w387:refnum<vi>)
    n228 = event shown="[3] <user event>: User Event" {
      selector: w405 -> [_ _ _ _ _ _ _ _ _ _ _ _ _ _]
      dyn-events: _ -> [_ _ _ _ _ _ _ _ _ _ _ _ _ _]
      timeout: _ -> [_ _ _ _ _ _ _ _ _ _ _ _ _ _]
      tunnel: [_ _ "plot (p)" _ _ _ "open (o)" _ _ _ _ _ _ _] -> _
      tunnel: w402 -> [_ w421 w511 w534 w698 w727 w746 _ _ _ _ _ w779 _]
      tunnel: w401 -> [_ w417 _ _ w710 _ _ _ _ _ _ _ _ _]
      tunnel: w400 -> [_ w416 _ w516 w706 _ _ _ _ _ _ _ _ _]
      tunnel: w399 -> [_ w415 _ w517 w702 _ _ _ _ _ _ _ _ _]
      tunnel: w398 -> [_ w411 _ w520 w711 w724 _ w748 w749 w751 w758 w769 _ _]
      tunnel: w397 -> [_ w418 _ w515 w699 w729 _ _ _ _ _ _ _ _]
      tunnel: w396 -> [_ _ _ w535 _ _ _ _ _ _ _ _ _ _]
      tunnel: "main folder" -> [_ _ _ w533 _ _ _ _ _ _ w759 w766 _ _]
      tunnel: w394 -> [_ _ _ w532 _ _ _ _ _ _ _ _ _ _]
      tunnel: w392 -> [_ w420 _ w525 w707 w725 _ _ _ _ _ _ _ w783]
      tunnel: w393 -> [_ w419 _ w524 w708 w726 _ _ _ _ _ _ _ _]
      tunnel: "temperature folder" -> [_ _ _ w530 _ _ _ _ _ _ _ _ w781 _]
      tunnel: w390 -> [_ _ _ w531 _ _ _ _ _ _ _ _ _ _]
      tunnel: "rotation set folder" -> [_ _ _ w529 _ _ _ _ _ _ _ _ _ _]
      tunnel: w388 -> [_ w410 _ w528 _ _ _ _ _ _ _ _ _ _]
      tunnel: w387 -> [_ w409 _ w527 _ _ _ _ _ _ _ _ w776 _]
      tunnel: w386 -> [_ w408 _ w518 w705 _ _ _ _ _ _ _ _ _]
      tunnel: w385 -> [_ w407 _ w513 _ _ _ _ _ _ _ _ w773 _]
      tunnel: w384 -> [_ _ _ _ _ _ _ _ _ _ _ w761 _ _]
      tunnel: w383 -> [_ _ _ w522 w704 _ _ _ _ _ _ _ _ _]
      tunnel: w382 -> [_ _ _ w521 w703 _ _ _ _ _ _ _ _ _]
      tunnel: w381 -> [_ _ _ w523 w701 _ _ _ _ _ _ _ _ _]
      tunnel: w380 -> [_ _ _ w526 w700 _ _ _ _ _ _ _ _ _]
      tunnel: w379 -> [_ w406 _ _ _ _ _ _ _ _ _ _ _ _]
      tunnel: w378 -> [_ _ _ w519 _ _ _ _ _ _ _ _ _ _]
      tunnel: w377 -> [_ _ _ w514 _ _ _ _ _ _ _ _ _ _]
      tunnel: w376 -> [_ _ _ w512 _ _ _ _ _ _ _ _ _ _]
      event Timeout {
        n229 = event-data() -> ()  [unwired: 1 in, 2 out]
      }
      event Key Down {
        n230 = event-data() -> ("Char"=w414:i16, "VKey"=w422:T2)  [unwired: 1 in]
        "Char" <- w414
        "VKey" <- w422
        n231 = Build Array(w414) -> (w413:i16[])
        n232 = Byte Array To String(unsigned byte array=w413) -> (string=w412:string)
        n233 = case shown="\"ASCII\", Default" w422 {
          selector: w422 -> [_ _ _ w478 _ _]
          tunnel: w414 -> [_ _ _ _ _ _]
          tunnel: w421 -> [w432 _ _ w476 w494 w502]
          tunnel: w420 -> [w431 _ _ _ _ _]
          tunnel: w419 -> [w430 _ _ w477 _ _]
          tunnel: w416 -> [_ w467 _ _ _ _]
          tunnel: w418 -> [_ w466 _ _ _ _]
          tunnel: w417 -> [w424 w465 _ _ _ _]
          tunnel: w415 -> [_ w464 _ _ _ _]
          tunnel: w412 -> [w429 _ _ _ _ _]
          tunnel: w411 -> [w428 _ _ w473 w491 _]
          tunnel: w410 -> [w427 _ _ _ w496 w504]
          tunnel: w409 -> [w426 _ _ _ w495 w503]
          tunnel: w408 -> [w423 w459 _ _ _ _]
          tunnel: w407 -> [w425 _ _ _ w493 w501]
          tunnel: w406 -> [_ w458 _ _ _ _]
          frame "ASCII", Default {
            n234 = case shown="\"c\"" w429 {
              tunnel: w432 -> [_ w433 w435 w437 w439 w441 w443 w445 w447 _]
              tunnel: w431 -> [_ _ _ _ _ _ _ _ _ w455]
              tunnel: w430 -> [_ _ _ _ _ _ _ _ _ w454]
              tunnel: w428 -> [_ _ _ _ _ _ _ _ _ _]
              tunnel: w427 -> [_ _ _ _ _ _ _ _ _ _]
              tunnel: w426 -> [_ _ _ _ _ _ _ _ _ _]
              tunnel: w425 -> [_ _ _ _ _ _ _ _ _ _]
              tunnel: w424 -> [_ _ _ _ _ _ _ _ _ w453]
              tunnel: w423 -> [_ _ _ _ _ _ _ _ _ w450]
              frame "0", Default {
              }
              frame "p" {
                # "p"
                n235 = Generate User Event(user event=w433, event data cluster="plot" ("event data")) -> ()  [unwired: 1 in, 2 out]
              }
              frame "o" {
                # "o"
                n236 = Generate User Event(user event=w435, event data cluster="read all angles" ("event data")) -> ()  [unwired: 1 in, 2 out]
              }
              frame "z" {
                n237 = Generate User Event(user event=w437, event data cluster="zoom out" ("event data")) -> ()  [unwired: 1 in, 2 out]
              }
              frame "y" {
                n238 = Generate User Event(user event=w439, event data cluster="save pink blue" ("event data")) -> ()  [unwired: 1 in, 2 out]
              }
              frame "r" {
                n239 = Generate User Event(user event=w441, event data cluster="remove offset" ("event data")) -> ()  [unwired: 1 in, 2 out]
              }
              frame "s" {
                n240 = Generate User Event(user event=w443, event data cluster="save slopes" ("event data")) -> ()  [unwired: 1 in, 2 out]
              }
              frame "R" {
                n241 = Generate User Event(user event=w445, event data cluster="re-read current angle" ("event data")) -> ()  [unwired: 1 in, 2 out]
              }
              frame " " {
                n242 = Generate User Event(user event=w447, event data cluster="plot all angles" ("event data")) -> ()  [unwired: 1 in, 2 out]
              }
              frame "c" {
                n243 = call "replace cursor - plot ref - V2.vi"("Plot ref in"=w453, "cursor action"=cursor_action."range") -> ()  [unwired: 15 in, 3 out]
                n244 = call "cursor window logic V2.vi"("cursor window action"=cursor_window_action."check", "cursor window in"=w454) -> ()  [unwired: 8 in, 2 out]
                n245 = call "cursor window logic V2.vi"("cursor window action"=cursor_window_action."check", "cursor window in"=w455) -> ()  [unwired: 8 in, 2 out]
                n246 = call "replace cursor - plot ref - V2.vi"("Plot ref in"=w450, "cursor index"=4, "cursor action"=cursor_action."range") -> ()  [unwired: 14 in, 3 out]
              }
            }
          }
          frame "Escape" {
            n247 = Build Array(w458, w467, w466, w465, w464, w459) -> (w463:refnum<vi>[])
            n248 = for {
              tunnel: w463 -> [w472] mode=indexing
              tunnel: [w471] -> w462
              tunnel: [w470] -> w460 mode=indexing
              n249 = property class="XYGraph (strict)"(reference=w472) -> (reference out=w470:refnum<vi>, "Palette Visible"=w471:bool)  [unwired: 1 in, 1 out]
            }
            n250 = Not(x=w462) -> (.not. x?=w461:bool)
            n251 = for {
              tunnel: w461 -> [w469]
              tunnel: w460 -> [w468] mode=indexing
              n252 = property class="XYGraph (strict)"(reference=w468, "Palette Visible"=w469) -> ()  [unwired: 1 in, 2 out]
            }
          }
          frame "Enter" {
          }
          frame "Up".."Right" {
            n253 = case shown="\"Down\"" w478 {
              tunnel: w477 -> [w479 w481 w483 w485 w487 w490]
              frame "Right", Default {
                n254 = call "cursor window logic V2.vi"("cursor window action"=cursor_window_action."move right", "cursor window in"=w479) -> ()  [unwired: 8 in, 2 out]
              }
              frame "Left" {
                n255 = call "cursor window logic V2.vi"("cursor window action"=cursor_window_action."move left", "cursor window in"=w481) -> ()  [unwired: 8 in, 2 out]
              }
              frame "PageUp" {
                n256 = call "cursor window logic V2.vi"("cursor window action"=cursor_window_action."skew up", "cursor window in"=w483) -> ()  [unwired: 8 in, 2 out]
              }
              frame "PageDown" {
                n257 = call "cursor window logic V2.vi"("cursor window action"=cursor_window_action."skew down", "cursor window in"=w485) -> ()  [unwired: 8 in, 2 out]
              }
              frame "Up" {
                n258 = call "cursor window logic V2.vi"("cursor window action"=cursor_window_action."broaden", "cursor window in"=w487) -> ()  [unwired: 8 in, 2 out]
              }
              frame "Down" {
                n259 = call "cursor window logic V2.vi"("cursor window action"=cursor_window_action."shrink", "cursor window in"=w490) -> ()  [unwired: 8 in, 2 out]
              }
            }
            n260 = Generate User Event(user event=w473, event data cluster="move all cursors" ("event data")) -> ()  [unwired: 1 in, 2 out]
            n261 = Generate User Event(user event=w476, event data cluster="fit one" ("event data")) -> ()  [unwired: 1 in, 2 out]
          }
          frame "PageUp" {
            w499 = hash_action_control."index forw" ("hash action")
            n262 = call "array -- smart enum.vi"("hash action"=w499, "hash"=w496) -> ()  [unwired: 5 in, 5 out]
            n263 = call "array -- smart enum.vi"("hash action"=w499, "hash"=w495) -> ("index OUT"=w498:i32)  [unwired: 5 in, 4 out]
            n264 = Generate User Event(user event=w494, event data cluster="plot one angle" ("event data")) -> ()  [unwired: 1 in, 2 out]
            n265 = Index Array(array=w493, index=w498) -> (element=w497:dbl)
            n266 = local write "current angle  index"(w498) -> ()
            n267 = Generate User Event(user event=w491, event data cluster="move red dots" ("event data")) -> ()  [unwired: 1 in, 2 out]
            n268 = local write "angle (deg)"(w497) -> ()
          }
          frame "PageDown" {
            w507 = hash_action_control."index back" ("hash action")
            n269 = call "array -- smart enum.vi"("hash action"=w507, "hash"=w504) -> ()  [unwired: 5 in, 5 out]
            n270 = call "array -- smart enum.vi"("hash action"=w507, "hash"=w503) -> ("index OUT"=w506:i32)  [unwired: 5 in, 4 out]
            n271 = Generate User Event(user event=w502, event data cluster="plot one angle" ("event data")) -> ()  [unwired: 1 in, 2 out]
            n272 = Index Array(array=w501, index=w506) -> (element=w505:dbl)
            n273 = local write "current angle  index"(w506) -> ()
            n274 = local write "angle (deg)"(w505) -> ()
          }
        }
      }
      event "plot (p)": Value Change {
        n275 = event-data() -> ()  [unwired: 1 in, 2 out]
        n276 = Generate User Event(user event=w511, event data cluster="plot" ("event data")) -> ()  [unwired: 1 in, 2 out]
      }
      event User Event {
        n277 = event-data() -> ("user event"=w536:string)  [unwired: 1 in]
        n278 = case shown="\"move red dots\"" w536 {
          tunnel: w516 -> [_ _ _ _ w658 _ _]
          tunnel: w517 -> [_ _ _ _ _ _ _]
          tunnel: w535 -> [_ _ _ _ _ _ _]
          tunnel: w534 -> [_ _ _ _ _ _ _]
          tunnel: w533 -> [_ w568 w597 _ _ _ _]
          tunnel: w532 -> [_ w567 _ _ _ _ _]
          tunnel: w520 -> [w540 w565 _ _ _ _ _]
          tunnel: w531 -> [w537 _ _ _ _ _ _]
          tunnel: w530 -> [_ _ w596 _ _ _ _]
          tunnel: w529 -> [w539 _ _ _ _ _ _]
          tunnel: w528 -> [_ _ w594 _ _ _ _]
          tunnel: w527 -> [_ _ w592 _ _ _ _]
          tunnel: w526 -> [_ _ _ _ _ w676 _]
          tunnel: w525 -> [_ _ _ w626 _ w675 _]
          tunnel: w524 -> [_ _ _ w627 _ w674 _]
          tunnel: w523 -> [_ _ _ _ _ w673 _]
          tunnel: w522 -> [_ _ _ _ w662 w672 _]
          tunnel: w521 -> [_ _ _ _ w648 w671 _]
          tunnel: w520 -> [_ _ _ _ _ _ _]
          tunnel: w519 -> [_ _ _ _ w661 _ _]
          tunnel: w518 -> [_ _ _ _ w660 _ _]
          tunnel: w517 -> [_ _ _ _ w659 _ _]
          tunnel: w515 -> [_ _ _ _ w657 _ _]
          tunnel: w514 -> [_ _ _ _ w653 _ _]
          tunnel: w513 -> [_ _ _ _ w652 _ _]
          tunnel: w512 -> [_ _ _ _ w650 _ _]
          frame "update list of temperatures" {
            (unwired) TRUE ("Numeric sort?")
            n279 = call "list - get folder names.vi"("regular expression"="\\s*([0-9\\.]+K\\S*)\\s*", "folder path"=w539) -> ("Array"=w543:string[], "OK"=w544:bool)  [unwired: 8 in]
            n280 = case shown="True" w544 {
              selector: w544 -> [w545 w559]
              tunnel: w537 -> [_ w553]
              tunnel: w543 -> [_ w555]
              tunnel: [w545 w559] -> w542
              tunnel: w539 -> [_ w558]
              frame False {
              }
              frame True {
                n281 = call "array -- smart enum.vi"("hash action"=hash_action_control."delete all", "hash"=w553) -> ("hash OUT"=w551:refnum<vi>)  [unwired: 5 in, 4 out]
                n282 = for {
                  tunnel: w555 -> [w561] mode=indexing
                  tunnel: hash_action_control."new" ("hash action") -> [w564]
                  shift-right: [w563] -> w550
                  shift-left: w551 -> [w562]
                  tunnel: [w560] -> w548 mode=indexing
                  n283 = Fract/Exp String To Number(string=w561) -> (number=w560:dbl)  [unwired: 3 in, 1 out]
                  n284 = call "array -- smart enum.vi"("hash action"=w564, "hash key"=w561, "hash"=w562) -> ("hash OUT"=w563:refnum<vi>)  [unwired: 4 in, 4 out]
                }
                n285 = local write "temperatures"(w548) -> ()
                n286 = call "array -- smart enum.vi"("hash action"=hash_action_control."check", "hash"=w550) -> ("index OUT"=w546:i32, "hash key OUT"=w549:string)  [unwired: 5 in, 3 out]
                n287 = Build Path(base path=w558, name or relative path=w549) -> (appended path=w557:path)
                n288 = local write "temperature folder"(w557) -> ()
                n289 = Index Array(array=w548, index=w546) -> (element=w547:dbl)
                n290 = local write "temperature (K)"(w547) -> ()
              }
            }
            n291 = Generate User Event(user event=w540, event data cluster="update list of angles" ("event data")) -> ()  [unwired: 1 in, 2 out]
            n292 = local write "folder --OK"(w542) -> ()
          }
          frame "update list of rotation sets" {
            (unwired) TRUE ("Numeric sort?")
            n293 = call "list - get folder names.vi"("folder path"=w568) -> ("Array"=w570:string[], "OK"=w571:bool)  [unwired: 9 in]
            n294 = case shown="True" w571 {
              selector: w571 -> [w572 w581]
              tunnel: w567 -> [_ w575]
              tunnel: w570 -> [_ w574]
              tunnel: [w572 w581] -> w569
              tunnel: w568 -> [_ w583]
              frame False {
              }
              frame True {
                n295 = call "array -- smart enum.vi"("hash action"=hash_action_control."delete all", "hash"=w575) -> ("hash OUT"=w577:refnum<vi>)  [unwired: 5 in, 4 out]
                n296 = for {
                  tunnel: w574 -> [w587] mode=indexing
                  tunnel: hash_action_control."new" ("hash action") -> [w586]
                  shift-right: [w585] -> w576
                  shift-left: w577 -> [w584]
                  n297 = call "array -- smart enum.vi"("hash action"=w586, "hash key"=w587, "hash"=w584) -> ("hash OUT"=w585:refnum<vi>)  [unwired: 4 in, 4 out]
                }
                n298 = call "array -- smart enum.vi"("hash action"=hash_action_control."check", "hash"=w576) -> ("hash key OUT"=w573:string)  [unwired: 5 in, 4 out]
                n299 = Build Path(base path=w583, name or relative path=w573) -> (appended path=w582:path)
                n300 = local write "rotation set folder"(w582) -> ()
              }
            }
            n301 = Generate User Event(user event=w565, event data cluster="update list of temperatures" ("event data")) -> ()  [unwired: 1 in, 2 out]
            n302 = local write "folder --OK"(w569) -> ()
          }
          frame "update list of angles" {
            (unwired) TRUE ("Numeric sort?")
            n303 = call "torque -- filename controller.vi"("filename action"=torque_--_filename_action."check") -> ("file name regexp"=w593:string)  [unwired: 6 in, 4 out]
            n304 = call "list - get file names - meta.vi"("match index"=2, "regular expression"=w593, "folder path"=w596) -> ("full name Array"=w590:string[], "match Array"=w591:string[], "OK"=w588:bool)  [unwired: 6 in]
            n305 = local write "folder --OK"(w588) -> ()
            n306 = case shown="True" w588 {
              tunnel: w594 -> [_ w605]
              tunnel: w591 -> [_ w603]
              tunnel: w597 -> [_ w615]
              tunnel: w592 -> [_ w609]
              tunnel: w590 -> [_ w608]
              frame False {
              }
              frame True {
                w606 = hash_action_control."delete all" ("hash action")
                n307 = call "array -- smart enum.vi"("hash action"=w606, "hash"=w609) -> ("hash OUT"=w611:refnum<vi>)  [unwired: 5 in, 4 out]
                n308 = call "array -- smart enum.vi"("hash action"=w606, "hash"=w605) -> ("hash OUT"=w604:refnum<vi>)  [unwired: 5 in, 4 out]
                n309 = for {
                  tunnel: hash_action_control."new" ("hash action") -> [w620]
                  shift-right: [w625] -> w610
                  shift-left: w611 -> [w624]
                  tunnel: w608 -> [w623] mode=indexing
                  shift-right: [w621] -> _
                  shift-left: w604 -> [w622]
                  tunnel: w603 -> [w619] mode=indexing
                  tunnel: [w618] -> w602 mode=indexing
                  tunnel: [0.0] -> w599 mode=indexing
                  tunnel: [T5 {"a"=0.0, "b"=0.0, "c"=0.0} ("parabola")] -> w598 mode=indexing
                  n310 = call "array -- smart enum.vi"("hash action"=w620, "hash key"=w623, "hash"=w624) -> ("hash OUT"=w625:refnum<vi>)  [unwired: 4 in, 4 out]
                  n311 = call "array -- smart enum.vi"("hash action"=w620, "hash key"=w619, "hash"=w622) -> ("hash OUT"=w621:refnum<vi>)  [unwired: 4 in, 4 out]
                  n312 = Fract/Exp String To Number(string=w619) -> (number=w618:dbl)  [unwired: 3 in, 1 out]
                }
                "sin2theta-fits" <- w598
                n313 = call "array -- smart enum.vi"("hash action"=hash_action_control."check", "hash"=w610) -> ("index OUT"=w601:i32, "hash key OUT"=w607:string)  [unwired: 5 in, 3 out]
                n314 = Build Path(base path=w615, name or relative path=w607) -> (appended path=w614:path)
                n315 = local write "file path"(w614) -> ()
                n316 = Index Array(array=w602, index=w601) -> (element=w600:dbl)
                n317 = local write "angles (deg)"(w602) -> ()
                n318 = local write "slopes"(w599) -> ()
                n319 = local write "angle (deg)"(w600) -> ()
              }
            }
          }
          frame "update other cursors" {
            n320 = call "cursor window logic V2.vi"("cursor window action"=cursor_window_action."check", "cursor window in"=w627) -> ("cursor window out"=w642:T4)  [unwired: 8 in, 1 out]
            n321 = Unbundle By Name(w642) -> ("left"=w639:dbl, "right"=w637:dbl)
            n322 = call "kim-read file -one.vi"("Numeric Control"=0, "container action"=container_action."get") -> ("Temperature (K) Array"=w634:dbl[], "time array"=w638:dbl[])  [unwired: 10 in, 6 out]
            n323 = Threshold 1D Array(2:w637, 3:w638) -> (0:w635:dbl)  [unwired: 1 in]
            n324 = Threshold 1D Array(2:w639, 3:w638) -> (0:w636:dbl)  [unwired: 1 in]
            n325 = Index Array(array=w634, index #1=w636, index #2=w635) -> (element #1=w633:dbl, element #2=w632:dbl)
            n326 = call "Q -- range multiplier -- real.vi"("factor"=1.0, "lower"=w633, "upper"=w632) -> ("center"=w628:dbl, "window"=w630:dbl)  [unwired: 5 in, 2 out]
            n327 = Absolute Value(x=w630) -> (abs(x)=w629:dbl)
            n328 = call "cursor window logic V2.vi"("cursor window action"=cursor_window_action."change cen&win", "window"=w629, "center"=w628, "cursor window in"=w626) -> ()  [unwired: 6 in, 2 out]
          }
          frame "move red dots" {
            w646 = cursor_action."write" ("cursor action")
            n329 = Bundle By Name(cluster=T12 {"temperature(K)"=0.0, "angle(deg)"=0.0} ("hash key"), "temperature(K)"=w662, "angle(deg)"=w648) -> (w663:T12)
            n330 = call "array -- find closest element.vi"("number"=w648, "Array"=w652) -> ("index"=w651:i32)  [unwired: 8 in, 1 out]
            n331 = call "torque - read all files V1.vi"("container action"=container_action."get", "hash key"=w663) -> ("torque -- hash value OUT"=w668:T15)  [unwired: 8 in, 1 out]
            n332 = Index Array(array=w650, index=w651) -> (element=w649:T5)
            n333 = local read "offset (deg)"() -> (w645:dbl)
            n334 = Unbundle By Name(w668) -> ("time (sec) array"=w667:dbl[], "field (T) array"=w666:dbl[], "SRS Vx (V) array"=w665:dbl[])
            n335 = Threshold 1D Array(2:w661, 3:w667) -> (0:w664:dbl)  [unwired: 1 in]
            n336 = local write "time (sec)"(w661) -> ()
            n337 = Index Array(array=w666, index=w664) -> (element=w655:dbl)
            n338 = Index Array(array=w665, index=w664) -> (element=w656:dbl)
            n339 = call "torque -- calc field div torque.vi"("angle offset"=w645, "parabola"=w649, "torque transformations"=w653, "angle"=w648, "torque"=w656, "field"=w655) -> ("transformed Y"=w654:dbl, "field out"=w647:dbl)  [unwired: 4 in]
            n340 = local write "Torque (a.u)"(w656) -> ()
            n341 = local write "field (T)"(w655) -> ()
            n342 = local write "current time index"(w664) -> ()
            n343 = call "replace cursor - plot ref - V2.vi"("Plot ref in"=w658, "new X"=w655, "new  Y"=w656, "cursor action"=w646) -> ()  [unwired: 13 in, 3 out]
            n344 = call "replace cursor - plot ref - V2.vi"("Plot ref in"=w659, "new X"=w655, "new  Y"=w656, "cursor action"=w646) -> ()  [unwired: 13 in, 3 out]
            n345 = call "replace cursor - plot ref - V2.vi"("Plot ref in"=w657, "new X"=w661, "cursor action"=w646) -> ()  [unwired: 14 in, 3 out]
            n346 = call "replace cursor - plot ref - V2.vi"("Plot ref in"=w660, "new X"=w647, "new  Y"=w654, "cursor action"=w646) -> ()  [unwired: 13 in, 3 out]
          }
          frame "move all cursors" {
            w685 = cursor_window_action."change cen&win" ("cursor window action")
            n347 = Bundle By Name(cluster=T12 {"temperature(K)"=0.0, "angle(deg)"=0.0} ("hash key"), "temperature(K)"=w672, "angle(deg)"=w671) -> (w677:T12)
            n348 = call "cursor window logic V2.vi"("cursor window action"=cursor_window_action."check", "cursor window in"=w674) -> ("cursor window out"=w696:T4)  [unwired: 8 in, 1 out]
            n349 = call "torque - read all files V1.vi"("container action"=container_action."get", "hash key"=w677) -> ("torque -- hash value OUT"=w693:T15)  [unwired: 8 in, 1 out]
            n350 = Unbundle By Name(w696) -> ("left"=w692:dbl, "right"=w690:dbl)
            n351 = Unbundle By Name(w693) -> ("time (sec) array"=w691:dbl[], "field (T) array"=w689:dbl[])
            n352 = Threshold 1D Array(2:w692, 3:w691) -> (0:w683:dbl)  [unwired: 1 in]
            n353 = Threshold 1D Array(2:w690, 3:w691) -> (0:w682:dbl)  [unwired: 1 in]
            n354 = Max & Min(x=w683, y=w682) -> (max(x,y)=w679:dbl, min(x,y)=w678:dbl)
            n355 = local write "right bound index"(w679) -> ()
            n356 = local write "left bound index"(w678) -> ()
            n357 = Index Array(array=w689, index #1=w679, index #2=w678) -> (element #1=w681:dbl, element #2=w680:dbl)
            n358 = Add(x=w681, y=w680) -> (x+y=w688:dbl)
            n359 = Subtract(x=w681, y=w680) -> (x-y=w684:dbl)
            n360 = Divide(x=w688, y=2.0) -> (x/y=w686:dbl)
            n361 = call "cursor window logic V2.vi"("cursor window action"=w685, "window"=w684, "center"=w686, "cursor window in"=w675) -> ()  [unwired: 6 in, 2 out]
            n362 = call "cursor window logic V2.vi"("cursor window action"=w685, "window"=w684, "center"=w686, "cursor window in"=w673) -> ()  [unwired: 6 in, 2 out]
            n363 = call "cursor window logic V2.vi"("cursor window action"=w685, "window"=w684, "center"=w686, "cursor window in"=w676) -> ()  [unwired: 6 in, 2 out]
          }
          frame "False", Default {
          }
        }
      }
      event "Plot: field vs time": Cursor Move {
        n364 = event-data() -> ("CursIdx"=w709:i32)  [unwired: 1 in]
        n365 = case shown="0" w709 {
          selector: w709 -> [w716 _ _]
          tunnel: w711 -> [w714 w719 _]
          tunnel: w710 -> [_ w722 _]
          tunnel: w708 -> [w717 _ _]
          tunnel: w707 -> [_ _ _]
          tunnel: w706 -> [_ _ _]
          tunnel: w705 -> [_ _ _]
          tunnel: w704 -> [_ _ _]
          tunnel: w703 -> [_ _ _]
          tunnel: w702 -> [_ _ _]
          tunnel: w701 -> [_ _ _]
          tunnel: w700 -> [_ _ _]
          tunnel: w699 -> [_ _ _]
          tunnel: w698 -> [w712 _ _]
          frame 1..3 {
            n366 = call "cursor window logic V2.vi"("CursIdx"=w716, "cursor window action"=cursor_window_action."cursor moves", "cursor window in"=w717) -> ()  [unwired: 7 in, 2 out]
            n367 = Generate User Event(user event=w714, event data cluster="move all cursors" ("event data")) -> ()  [unwired: 1 in, 2 out]
            n368 = Generate User Event(user event=w712, event data cluster="fit one" ("event data")) -> ()  [unwired: 1 in, 2 out]
          }
          frame 0 {
            n369 = call "replace cursor - plot ref - V2.vi"("Plot ref in"=w722, "cursor action"=cursor_action."read") -> ("read X"=w721:dbl)  [unwired: 15 in, 2 out]
            n370 = local write "time (sec)"(w721) -> ()
            n371 = Generate User Event(user event=w719, event data cluster="move red dots" ("event data")) -> ()  [unwired: 1 in, 2 out]
          }
          frame -1, Default {
          }
        }
      }
      event "Plot: temp vs time": Cursor Move {
        n372 = event-data() -> ("CursIdx"=w728:i32)  [unwired: 1 in]
        n373 = case shown="1..3, Default" w728 {
          selector: w728 -> [w733 _]
          tunnel: w729 -> [_ w740]
          tunnel: w727 -> [_ w735]
          tunnel: w726 -> [w732 _]
          tunnel: w725 -> [_ _]
          tunnel: w724 -> [w730 _]
          frame 1..3, Default {
            (unwired) container_action."get" ("container action")
            (unwired) 0 ("Numeric Control")
            n374 = call "cursor window logic V2.vi"("CursIdx"=w733, "cursor window action"=cursor_window_action."cursor moves", "cursor window in"=w732) -> ()  [unwired: 7 in, 2 out]
            n375 = Generate User Event(user event=w730, event data cluster="update other cursors" ("event data")) -> ()  [unwired: 1 in, 2 out]
          }
          frame 0 {
            n376 = call "replace cursor - plot ref - V1.vi"("action"=enum16{"", "read", "write"}."read", "Plot ref in"=w740) -> ("read X"=w742:dbl)  [unwired: 7 in, 2 out]
            n377 = call "kim-read file -one.vi"("Numeric Control"=0, "container action"=container_action."get") -> ("time array"=w738:dbl[])  [unwired: 10 in, 7 out]
            n378 = Threshold 1D Array(2:w742, 3:w738) -> (0:w741:dbl)  [unwired: 1 in]
            n379 = local write "current angle  index"(w741) -> ()
            n380 = local write "time (sec)"(w742) -> ()
            n381 = Generate User Event(user event=w735, event data cluster="update cursor -- from temperature plot" ("event data")) -> ()  [unwired: 1 in, 2 out]
          }
        }
      }
      event "open (o)": Value Change {
        n382 = event-data() -> ()  [unwired: 1 in, 2 out]
        n383 = Generate User Event(user event=w746, event data cluster="read all angles" ("event data")) -> ()  [unwired: 1 in, 2 out]
      }
      event "rotation set": Mouse Enter {
        n384 = event-data() -> ()  [unwired: 1 in, 4 out]
        n385 = Generate User Event(user event=w748, event data cluster="update list of rotation sets" ("event data")) -> ()  [unwired: 1 in, 2 out]
      }
      event "temperature": Mouse Enter {
        n386 = event-data() -> ()  [unwired: 1 in, 4 out]
        n387 = Generate User Event(user event=w749, event data cluster="update list of temperatures" ("event data")) -> ()  [unwired: 1 in, 2 out]
      }
      event "angle": Mouse Enter {
        n388 = event-data() -> ()  [unwired: 1 in, 4 out]
        n389 = Generate User Event(user event=w751, event data cluster="update list of angles" ("event data")) -> ()  [unwired: 1 in, 2 out]
      }
      event "rotation set": Value Change {
        n390 = event-data() -> ("CtlRef"=w755:refnum<vi>)  [unwired: 1 in]
        n391 = call "array -- smart enum.vi"("hash action"=hash_action_control."check", "hash"=w755) -> ("hash key OUT"=w753:string)  [unwired: 5 in, 4 out]
        n392 = Build Path(base path=w759, name or relative path=w753) -> (appended path=w756:path)
        n393 = local write "temperature folder"(w756) -> ()
        n394 = Generate User Event(user event=w758, event data cluster="update list of temperatures" ("event data")) -> ()  [unwired: 1 in, 2 out]
      }
      event "temperature": Value Change {
        n395 = event-data() -> ("CtlRef"=w764:refnum<vi>)  [unwired: 1 in]
        n396 = call "array -- smart enum.vi"("hash action"=hash_action_control."check", "hash"=w764) -> ("index OUT"=w762:i32, "hash key OUT"=w763:string)  [unwired: 5 in, 3 out]
        n397 = Index Array(array=w761, index=w762) -> (element=w760:dbl)
        n398 = Build Path(base path=w766, name or relative path=w763) -> (appended path=w767:path)
        n399 = local write "temperature (K)"(w760) -> ()
        n400 = local write "temperature folder"(w767) -> ()
        n401 = Generate User Event(user event=w769, event data cluster="update list of angles" ("event data")) -> ()  [unwired: 1 in, 2 out]
      }
      event "angle": Value Change {
        n402 = event-data() -> ("CtlRef"=w777:refnum<vi>)  [unwired: 1 in]
        n403 = call "array -- smart enum.vi"("hash action"=hash_action_control."check", "hash"=w777) -> ("index OUT"=w770:i32)  [unwired: 5 in, 4 out]
        n404 = call "array -- smart enum.vi"("hash action"=hash_action_control."index set", "index IN"=w770, "hash"=w776) -> ("index OUT"=w772:i32, "hash key OUT"=w774:string)  [unwired: 4 in, 3 out]
        n405 = local write "current angle  index"(w770) -> ()
        n406 = Index Array(array=w773, index=w772) -> (element=w771:dbl)
        n407 = Build Path(base path=w781, name or relative path=w774) -> (appended path=w782:path)
        n408 = local write "angle (deg)"(w771) -> ()
        n409 = local write "file path"(w782) -> ()
        n410 = Generate User Event(user event=w779, event data cluster="plot one angle" ("event data")) -> ()  [unwired: 1 in, 2 out]
      }
      event "Plot: torque -- all angles": Cursor Move {
        n411 = event-data() -> ("CursIdx"=w784:i32)  [unwired: 1 in, 3 out]
        n412 = call "cursor window logic V2.vi"("CursIdx"=w784, "cursor window action"=cursor_window_action."cursor moves", "cursor window in"=w783) -> ()  [unwired: 7 in, 2 out]
      }
    }
    n413 = Wait (ms)(milliseconds to wait=u32 1) -> ()  [unwired: 1 out]
  }
  n414 = control-ref of="timer  \"update\""() -> (w56:refnum<vi>)
  n415 = call "slider timer .vi"("action"=countdown_control."start", "timer ref"=w56) -> ("timer out"=w55:refnum<vi>)  [unwired: 7 in, 2 out]
  n416 = while {
    shift-right: [w790] -> _
    shift-left: w55 -> [w791]
    tunnel: w54 -> [w787]
    stop <- FALSE stop-if-true
    n417 = case shown="\"timer ON\", Default" "Tab: timer" {
      tunnel: w791 -> [w795 w799]
      tunnel: [w794 w799] -> w790
      tunnel: w787 -> [w792 _]
      frame "timer ON", Default {
        n418 = call "slider timer .vi"("action"=countdown_control."check", "timer ref"=w795) -> ("tic"=w793:bool, "timer out"=w794:refnum<vi>)  [unwired: 7 in, 1 out]
        n419 = case shown="True" w793 {
          tunnel: w792 -> [_ w797]
          frame False {
          }
          frame True {
            n420 = Generate User Event(user event=w797, event data cluster="read file" ("event data")) -> ()  [unwired: 1 in, 2 out]
          }
        }
      }
      frame "timer OFF" {
      }
    }
    n421 = Wait (ms)(milliseconds to wait=u32 123) -> ()  [unwired: 1 out]
  }
